vi "UHR-Fleezers Control (fpga) - 11.7.1UCBMeng4RG3.vi"() -> ()   [LabVIEW 2014]
doc: "UHR-Fleezers Instrument Control Code (fpga)"
uses:
  <vilib>/Platform/TimedLoop/XDataNode/timing_clust.ctl
  <vilib>/Platform/TimedLoop/XDataNode/nitl_modes.ctl
  <vilib>/Platform/TimedLoop/XDataNode/wakeup.ctl
  <vilib>/rvi/Emulation/niFpgaGetClockAttributes.vi
  <vilib>/rvi/Emulation/niFpgaSctlEmulationGetInTimedLoop.vi
  <vilib>/rvi/Emulation/niFpgaEmulationReportErrorSimple.vi
  <vilib>/rvi/Emulation/niFpgaProcessEmulError.vi
  <vilib>/rvi/eio/common/nirviEmuTemplateMethod_errors.vi
  <vilib>/rvi/Emulation/niFpgaCriticalErrorInLSC.vi
  <vilib>/rvi/interface/RandomDataEmulation/niFpgaRandomDataHandleErrors.vi
  <vilib>/eio/EIONode/EIONode.xnode
  <vilib>/eio/EIOMethodNode/EIOMethodNode.xnode
  <vilib>/rvi/DataTransferAndStorage/Container/XNode/niFpgaContainer.xnode
  <vilib>/rvi/interface/RandomDataEmulation/nirviRandomDataFpgaReadWriteTemplate.vi
  <vilib>/addons/control/pid/fpga.llb/XNode/niFpgaPID.xnode
  <vilib>/Platform/TimedLoop/XDataNode/XDataNode.xnode
  <vilib>/Platform/TimedLoop/XDataNode/XDNodeRunTimeDep.lvlib
panel:
  in  "Tab Control":T1(tab)=enum."Force FB"
  in  "Set 3":bool
  in  "Set 2":bool=TRUE
  in  "Set 1":bool=TRUE
  in  "Trap Pos to FIFO":bool
  in  "N of AI1 Int Acq Sets":i16=2 min=1 max=3 step=1
  out "AI Late Counter":u8
  in  "ai count":u16=400
  in  "+ phase":bool
  in  "Phase count adjustment":i16
  out "Relative phase":i16
  in  "AI to FIFO":bool
  out "BD1 Frequency Out 1":u64
  out "BD1 Frequency Out 2":u64
  out "Trap Pos FIFO Timeout":u16
  out "Trap AI FIFO Timeout":u16
  in  "Trap FIFO Set Timeout":i32
  in  "Tab Control 2":T2(tab)
  in  "FB Offset":u16
  in  "FB Multi Factor":i16
  in  "Dynamic FB (Ronen)":bool
  in  "Negate Intensity FB":bool
  in  "RD":bool
  in  "FB1 output high":i16=3000
  in  "FB1 output low":i16
  in  "D1":i16
  in  "I1":i16=5
  in  "P1":i16=10
  in  "Swap F1 and F2":bool
  in  "Cont. Scan":bool
  in  "Abort scan":bool
  in  "Cycles per step":u64
  in  "Scan BD":bool
  in  "Number of scans":u16
  in  "Scan steps":u64
  in  "Scan freq.  increment":i64
  out "Scanning":bool
  in  "Start scan":bool
  in  "OSK Bd 1":bool
  in  "Reset Bd 1":bool
  in  "PMODE":bool
  in  "Direct RF Box \nCommunication":bool
  in  "Data BD 2":u8 format="%08b"
  in  "Data BD 1":u8 format="%08b"
  in  "Address":u8 format="%02x"
  in  "Update Data":bool
  in  "FPGA Controls\n RF Box":bool
  in  "Number Interlace Cycles":u8=2 min=1 max=3
  in  "Interlace Off Parameters":u8=1 min=1 max=3
  in  "Interlace ON/OFF":bool
  out "DIO Relative phase":i16
  in  "Phase count adjustment (DIO)":i16
  in  "+ phase (DIO)":bool
  out "DIO Late Counter":u8
  in  "DIO count 1 (ticks)":u16=400
  in  "DIO count 2 (ticks)":u16=400
  in  "DIO count 3 (ticks)":u16=400
  out "AI2 Y Sum Set 2":i16
  out "AI2 Y Sum Set 1":i16
  in  "FB Setpoint Set 1":i16 min=0 step=1
  in  "FB Reset Set 1":bool
  in  "FB On/Off Set 1":bool
  in  "FB Reset Set 2":bool
  in  "FB On/Off Set 2":bool
  in  "FB Setpoint Set 2":i16 min=0 step=1
  out "Scan I":u64
  in  "Amp switch delay":u8=5
  in  "XY phase ext loop method":bool
  in  "BD 2 Amplitude 1":u16
  in  "BD 1 Amplitude 1":u16
  in  "BD 2 Frequency 1":u64
  in  "BD 1 Frequency 1":u64
  in  "BD 2 Amplitude 2":u16
  in  "BD 1 Amplitude 2":u16
  in  "BD 2 Frequency 2":u64
  in  "BD 1 Frequency 2":u64
  in  "BD 2 Amplitude 3":u16
  in  "BD 1 Amplitude 3":u16
  in  "BD 2 Frequency 3":u64
  in  "BD 1 Frequency 3":u64
  in  "BD 1 Delay (ticks)":u8
  in  "BD 2 Delay (Ticks)":u8 caption="Count(Ticks)"
  in  "Next trap write delay (ticks)":u8 caption="Count(Ticks)"
  in  "Trap 1 osc enable":bool
  in  "Trap 2 osc enable":bool
  in  "FB Min frequency":u64
  in  "FB Max Frequency":u64
  in  "Dynamic Force FB (Ronen)":bool
  in  "FB2 output high":fxp<+/-,16,1>=0.999969482421875
  in  "FB2 output low":fxp<+/-,16,1>=-1.0
  in  "P2":fxp<+/-,16,8> format="%.11g"
  in  "I2":fxp<+/-,16,8>=10.0 format="%.11g"
  in  "D2":fxp<+/-,16,8> format="%.11g"
  in  "Negate Diff?":bool
  in  "Diff FB Measurement?":bool
  in  "FB Trig Integrate":u32=1
  out "TTrig?":bool
  in  "TTrig Negate Pos":bool=TRUE
  out "Trap Pos FB Int Signal":fxp<+/-,24,9> format="%.18g"
  out "Trap Pos FB Int-Norm Signal":fxp<+/-,16,1> format="%.16g"
  in  "FPGA TTrig Thresh":i64
  in  "FPGA Trap Trig":bool
  out "Trap Pos FB Action":i64
  in  "Trap Pos. FB Offset Factor":i64
  in  "Trap Pos. FB Mult Factor":i64=2
  in  "Trap Pos. FB Reset":bool
  in  "Trap Pos FB Monitor T1 or T2":bool
  in  "AI1 X Scale":u16
  in  "Trap Pos FB Int Count":u16=100
  in  "Trap Pos FB Negate Action":bool
  out "AI1 X Set 2":fxp<+/-,16,1>
  out "AI1 X Set 1":fxp<+/-,16,1>
  in  "Trap Pos. FB SP":fxp<+/-,16,1>
  in  "Force feedback":bool
  out "TTrig Sig":i64
  out "TTrig Fin Thresh":i64
  in  "1D or 2D Scan?":bool
  in  "Abort scan (MCL)":bool
  in  "MCL Scan Axis":bool
  in  "Cont. Scan (MCL)":bool
  out "Scan I (MCL)":u64
  in  "Number of scans (MCL)":u16
  out "Scanning MCL":bool
  in  "Scan steps (MCL)":u64
  in  "Cycles per step (MCL)":u64
  in  "Scan freq.  increment (MCL)":i16
  in  "Start scan (MCL)":bool
  in  "AO2":i16
  in  "AO1":i16
  out "MCL Late Counter":u8
  in  "MCL count":u32=800
  out "MCL Relative Phase":i16
  in  "Phase count adjustment (MCL)":i16
  in  "+ phase (MCL)":bool
  out "APD2 int gate":bool
  out "APD3 out state":bool
  in  "APD Gate Operating Mode":u8 max=2 step=1
  in  "Invert APD Gate":bool
  in  "APD Gate OFF Count":u16=100
  in  "APD Gate ON Count":u16=300
  out "APD 1 Gate Late Counter":u8
  out "APD 1 Gate Relative Phase":i16
  in  "Phase count adjustment (APD 1 Gate)":i16
  in  "+ phase (APD 1 Gate)":bool
  out "APD 2 Counts 0":u32
  out "APD 2 Counts 1":u32
  out "APD 1 Counts 0":u32
  out "APD 1 Counts 1":u32
  out "APD1 out state":bool
  in  "APD AO scale factor":i16=1
  in  "APD to FIFO":bool
  in  "APD Acq Rate Count":u32=20000000
  out "APD Acq Late Counter":u8
  out "APD Acq Relative Phase":i16
  in  "Phase Count Adjustment (APD Acq)":i16
  in  "+ phase (APD Acq)":bool
  in  "Phase count adjustment (APD 2 Gate)":i16
  out "APD 2 Gate Late Counter":u8
  out "APD 2 Gate Relative Phase":i16
  in  "+ phase (APD 2 Gate)":bool
  out "APD2 out state":bool
  out "APD 3 Counts 0":u32
  out "APD 3 Counts 1":u32
  out "APD 3 Gate Late Counter":u8
  in  "Phase count adjustment (APD 3 Gate)":i16
  out "APD 3 Gate Relative Phase":i16
  in  "+ phase (APD 3 Gate)":bool
  out "APD1 int gate":bool
  out "APD3 int gate":bool
  in  "D3":i16
  in  "I3":i16=5
  in  "P3":i16=10
  in  "Green Filter Flipper":bool
  in  "Green FB Count":u16=1200
  out "Green Late Counter":u8
  out "Green FB Relative Phase":i16
  in  "Phase count adjustment (Green FB)":i16=10
  in  "+ phase (Green FB)":bool
  out "Green FB Sum":i16
  in  "Green int current ON count adj":u16=150
  in  "Current Out":u16=30000
  in  "Green FB On/Off":bool
  in  "Green FB Setpoint":i16=250 min=0 step=1
  in  "Green FB Reset":bool
  in  "Operating Mode 2":u8=2 max=2 step=1
  in  "Invert GI 2":bool
  in  "Green interlace OFF count 2":u16=900
  in  "Green interlace ON count 2":u16=300
  out "GI Late Counter 2":u8
  out "GI Relative phase 2":i16
  in  "Phase count adjustment (GI) 2":i16=20
  in  "+ phase (GI) 2":bool
  in  "Green interlace OFF count":u16=100
  out "GI Relative phase":i16
  in  "Phase count adjustment (GI)":i16
  in  "+ phase (GI)":bool
  in  "Green interlace ON count":u16=300
  out "GI Late Counter":u8
  in  "Invert GI":bool
  in  "Operating Mode":u8 max=2 step=1
  in  "+ phase (RI)":bool
  out "RI Relative phase":i16
  out "RI Late Counter":u8
  in  "Red interlace ON count":u16=300
  in  "Red interlace OFF count":u16=100
  in  "Invert RI":bool
  in  "Red Laser Operating Mode":u8 max=2 step=1
  in  "Phase count adjustment (RI)":i16
  out "Red FB Intensity":i16
  in  "RI Current Out":u16=30000
  in  "Red FB On/Off":bool
  in  "D4":i16
  in  "I4":i16=5
  in  "P4":i16=10
  in  "Red FB Setpoint":i16=250 min=0 step=1
  in  "Red FB Reset":bool
  in  "RI Operating Mode 2":u8=2 max=2 step=1
  in  "Invert RI 2":bool
  in  "Phase count adjustment (BI AO)":i16=20
  in  "Blue current ON count adj (AO)":u16=150
  in  "BI Current Out":i16=30000
  in  "Blue FB On/Off":bool
  in  "D5":i16
  in  "I5":i16=5
  in  "P5":i16=10
  in  "Blue FB Setpoint":i16=250 min=0 step=1
  in  "Blue FB Reset":bool
  in  "BI Operating Mode (AO)":u8=2 max=2 step=1
  in  "Invert BI (AO)":bool
  in  "Blue OFF count (AO)":u16=900
  in  "Blue ON count (AO)":u16=300
  out "BI Late Counter (AO)":u8
  out "BI Relative phase (AO)":i16
  in  "+ phase (BI AO)":bool
  in  "Phase count adjustment (BI D)":i16
  in  "Blue Laser Operating Mode (D)":u8 max=2 step=1
  in  "Invert BI (D)":bool
  in  "Blue interlace OFF count (D)":u16=100
  in  "Blue interlace ON count (D)":u16=300
  out "Blue Late Counter (D)":u8
  out "BI Relative phase (D)":i16
  in  "+ phase (BI D)":bool
  out "Blue Intensity":i16
  # "Only one of these can be on\nat a time:"
  # "Raster Scan AOD"
  # "1 (X)"
  # "2 (Y)"
  # "IR Intensity Feedback (RF BD 1)"
  # "FB Gains Set 1"
  # "FB output range 1"
  # "False is usual, True is external loop method"
  # "Parameters if using the external RF switching loop"
  # "Parameters if using the usual internal RF switching method"
  # "FB Triggering Excitation Laser"
  # "Trap Pos. FB Gains"
  # "Trap Pos. FB Range"
  # "AO1 (Y)"
  # "2D"
  # "1D"
  # "AO2 (X)"
  # "APD AO for aligning"
  # "Detection Loop"
  # "Green fluorescent laser digital gate interlacing loop"
  # "0 Forced ON\n1 Forced OFF\n2 Interlacing"
  # "Green FB Gains"
  # "Red fluorescent laser digital gate interlacing loop"
  # "Detection Loop"
  # "0 Forced ON\n1 Forced OFF\n2 Interlacing"
  # "Analog/FB Control Loop\n(Disabled)"
  # "Digital Control Loop"
  # "Blue laser intensity reading"
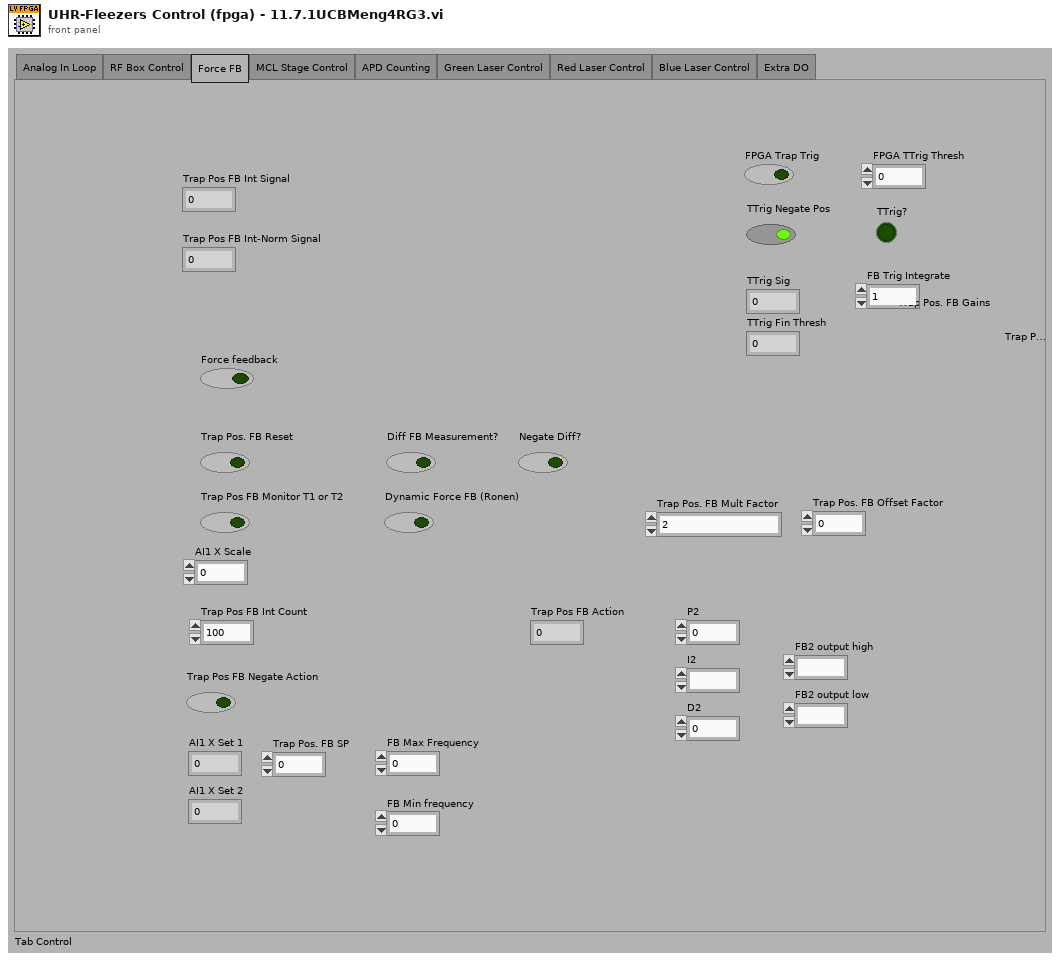
[diagram p1: front panel]
types:
  T1 = enum32{"Analog In Loop", "RF Box Control", "Force FB", "MCL Stage Control", "APD Counting", "Green Laser Control", "Red Laser Control", "Blue Laser Control", "Extra DO"}
  T2 = enum32{"Controls", "Interlacing Frequency and Amplitude Values", "Oscillate trap from memory"}
  T3 = typedef "XDNodeRunTimeDep.lvlib/timing_clust.ctl" = cluster{"Expected End [f-1]":u64, "Actual End [f-1]":u64, "Finished Late? [f-1]":bool, "Expected End [i-1]":u64, "Actual End [i-1]":u64, "Finished Late? [i-1]":bool, "Expected Start [i]":u64, "Actual Start [i]":u64, "Expected Start [f]":u64, "Actual Start [f]":u64, "Source Name":string, "Structure Name":string, "Period":i64, "Deadline":i64, "Offset":i64, "Start":i64, "Priority":i32, "Timeout":i32, "Mode":T4, "Wakeup Reason":T5, "Error":errorcluster, "Source Type":string, "Secondary Source Type":string, "Global End Time":u64, "Global Start Time":u64, "Frame Duration":u64, "Iteration Duration":u64, "Assigned CPU":i32, "I/O Scan Engine Mode":u32}
  T4 = typedef "XDNodeRunTimeDep.lvlib/nitl_modes.ctl" = enum32{"No Change", "Process missed periods, maintain original phase", "Discard missed periods, maintain original phase", "Process missed periods, ignore original phase", "Discard missed periods, ignore original phase"}
  T5 = typedef "XDNodeRunTimeDep.lvlib/wakeup.ctl" = enum32{"Normal", "Aborted", "Asynchronous wakeup", "Timing source error", "Timed loop error", "Timeout"}
  T6 = cluster{"proportional gain (Kc)":i16, "integral gain (Kc*Ts/Ti)":i16, "derivative gain (Kc*Td/Ts)":i16}
  T7 = cluster{"FB1 output high":i16, "FB1 output low":i16}
  T8 = cluster{"P2":fxp<+/-,16,8>, "I2":fxp<+/-,16,8>, "D2":fxp<+/-,16,8>}
  T9 = cluster{"FB2 output high":fxp<+/-,16,1>, "FB2 output low":fxp<+/-,16,1>}
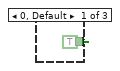
[diagram p2: hidden frame]
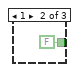
[diagram p3: hidden frame]
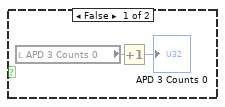
[diagram p6: hidden frame]
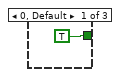
[diagram p8: hidden frame]
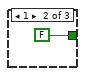
[diagram p9: hidden frame]
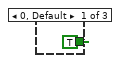
[diagram p10: hidden frame]
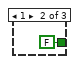
[diagram p11: hidden frame]
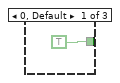
[diagram p13: hidden frame]
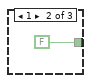
[diagram p14: hidden frame]
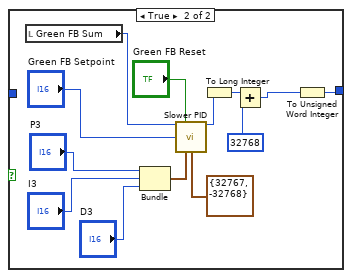
[diagram p17: hidden frame]
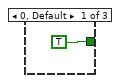
[diagram p18: hidden frame]
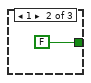
[diagram p19: hidden frame]
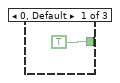
[diagram p20: hidden frame]
diagram:
  w6 = u16 0
  w7 = FALSE
  w5 = FALSE
  # "timing array current index"
  # "timing array"
  # "timing counter (phase adjusted here)"
  # "late counter"
  n1 = flat-sequence "FPGA initialization to do before running any of the loops" {
    tunnel: [u16 0 ("DIO count 3 (ticks)")] -> w4
    tunnel: [w15] -> _
    frame #0 {
      w14 = FALSE ("Enable")
      # "BD 2 (Y)"
      # "BD 1 (X)"
      # "Start up expansion chassis early\nto avoid delays later"
      # "This pin controls udclk on the RF boards.\nWhen initially configuring the boards, this pin needs to be\nconfigured as a high impedance input.  Later it will be switched\nto an output."
      # "Initial setting of DIO data and \naddress to low (before reset).  \nThis needs to happen before the other\ncontrol method loops execute."
      n2 = xnode "FPGA I/O Node"("Chassis2/Mod1/AO0"=u16 0 ("Chassis2/Mod4/AO0")) -> ("Chassis2/Mod2/AI0"=w15:i16)  [unwired: 2 in, 2 out]
      n3 = xnode "FPGA I/O Method Node"("Enable"=w14) -> ()  [unwired: 1 in, 1 out]
      n4 = xnode "FPGA I/O Method Node"("Enable"=w14) -> ()  [unwired: 1 in, 1 out]
      n5 = xnode "FPGA I/O Node"("Connector1/DIO0"=FALSE, "Connector1/DIO1"=FALSE, "Connector1/DIO2"=FALSE, "Connector1/DIO3"=FALSE, "Connector1/DIO4"=FALSE, "Connector1/DIO5"=FALSE, "Connector1/DIO6"=FALSE, "Connector1/DIO7"=FALSE, "Connector1/DIO8"=FALSE, "Connector1/DIO9"=FALSE, "Connector1/DIO10"=FALSE, "Connector1/DIO11"=FALSE, "Connector1/DIO12"=FALSE, "Connector1/DIO13"=FALSE, "Connector1/DIO15"=FALSE, "Connector1/DIO20"=FALSE, "Connector1/DIO21"=FALSE, "Connector1/DIO22"=FALSE, "Connector1/DIO23"=FALSE, "Connector1/DIO24"=FALSE, "Connector1/DIO25"=FALSE, "Connector1/DIO26"=FALSE, "Connector1/DIO27"=FALSE, "Connector1/DIO14"=FALSE) -> ()  [unwired: 24 in, 24 out]
    }
  }
  n6 = local read "AO1"() -> (w12:i16)
  n7 = local read "AO2"() -> (w11:i16)
  n8 = node-c288() -> (w10:T3)  [unwired: 1 in]
  n9 = disable-structure shown="Disabled" {
    disable-tunnel: w4 -> [w42 _]
    frame Disabled {
      n10 = while "Excitation laser intensity feedback measurement (all lasers)" {
        shift-right: [w43] -> _
        shift-left: w42 -> [w48]
        stop <- FALSE stop-if-true
        n11 = flat-sequence {
          tunnel: w48 -> [w50]
          tunnel: [w51] -> w46
          tunnel: [w50] -> w44
          tunnel: [w57] -> w47
          tunnel: w46 -> [w57]
          tunnel: [w56] -> w45
          tunnel: w44 -> [w56]
          tunnel: [w69] -> w43
          tunnel: w47 -> [w80]
          tunnel: w45 -> [w77]
          frame #0 {
            n12 = call "Loop Timer9"("Count(Ticks)"=w50) -> ("Tick Count(Ticks)"=w51:u16)
          }
          frame #1 {
            # "Design note:\n\nAll lasers need to be measured at the same \ntime because the AI expansion module\ncannot independently time the measurements\nwithin our requirements: their is dead time.\n\nThis probably wouldn't be an issue with the built\nin AI on the fpga board itself."
            n13 = xnode "FPGA I/O Node"("Connector1/DIO35"=TRUE) -> ("Chassis2/Mod2/AI2"=→"Blue Intensity":i16, "Chassis2/Mod2/AI1"=→"Red FB Intensity":i16, "Chassis2/Mod2/AI0"=→"Green FB Sum":i16)  [unwired: 4 in, 4 out]
          }
          frame #2 {
            n14 = feedback-in #1(w80) -> ()
            n15 = feedback #1(w80) -> (w79:u16)
            n16 = Subtract(x=w80, y=w79) -> (x-y=w78:u16)
            n17 = xnode "FPGA I/O Node"("Connector1/DIO35"=FALSE) -> ()  [unwired: 1 in, 1 out]
            n18 = Subtract(x=w78, y=w77) -> (x-y=w59:u16)
            n19 = Subtract(x="Green FB Count", y=w59) -> (x-y=w73:u16)
            n20 = Number To Boolean Array(number=w59) -> (Boolean array=w60:bool[])
            n21 = Or Array Elements(Boolean array=w60) -> (logical OR=w58:bool)
            n22 = Boolean To (0,1)(Boolean="+ phase (Green FB)") -> (0, 1=w71:i16)
            n23 = Boolean To (0,1)(Boolean=w58) -> (0, 1=w65:i16)
            n24 = Multiply(x=w71, y="Phase count adjustment (Green FB)") -> (x*y=w66:i16)
            n25 = Add(x=w73, y=w66) -> (x+y=w69:u16)
            n26 = To Unsigned Byte Integer(number=w65) -> (unsigned 8bit integer=w62:u8)
            n27 = feedback #2(i16 0) -> (w68:i16)
            n28 = Subtract(x=w68, y=w66) -> (x-y=w67:i16)
            "Green FB Relative Phase" <- w67
            n29 = feedback-in #2(w67) -> ()
            n30 = feedback #3(u8 0) -> (w63:u8)
            n31 = Add(x=w62, y=w63) -> (x+y=w61:u8)
            "Green Late Counter" <- w61
            n32 = feedback-in #3(w61) -> ()
          }
        }
      }
    }
    frame Enabled {
    }
  }
  n33 = To Unsigned Long Integer(number=w4) -> (unsigned 32bit integer=w8:u32)
  n34 = timed-loop "RF box board DIO control: control bits" {
    timing: w10 -> [_]
    timing-out: [_] -> w9
    tunnel: [w83] -> _
    tunnel: w4 -> [w83]
    stop <- FALSE stop-if-true
    n35 = xnode "FPGA I/O Node"("Connector1/DIO16"="RD", "Connector1/DIO17"="PMODE", "Connector1/DIO18"="OSK Bd 1", "Connector1/DIO19"="Reset Bd 1", "Connector0/DIO3"="Green Filter Flipper") -> ()  [unwired: 5 in, 5 out]
  }
  n36 = while "RF box board direct communication loop" {
    tunnel: w4 -> [_]
    stop <- FALSE stop-if-true
    n37 = case "Whether to use direct communication method (only use one method at a time)" shown="True" "Direct RF Box \nCommunication" {
      frame False {
      }
      frame True {
        n38 = case shown="True" "Update Data" {
          frame False {
          }
          frame True {
            n39 = flat-sequence {
              frame #0 {
                n40 = First Call?() -> (First Call?: T/F=w93:bool)
                n41 = case shown="True" w93 {
                  frame False {
                  }
                  frame True {
                    # "If first time data updated, be sure to set WR high\nbefore setting data and address bits."
                    n42 = flat-sequence {
                      frame #0 {
                        n43 = xnode "FPGA I/O Node"("Connector1/DIO15"=TRUE) -> ()  [unwired: 1 in, 1 out]
                      }
                      frame #1 {
                        n44 = call "Wait"("Count(Ticks)"=u8 40 ("DO Delay 3 (Ticks)")) -> ()  [unwired: 1 out]
                      }
                    }
                  }
                }
              }
              frame #1 {
                n45 = Number To Boolean Array(number="Address") -> (Boolean array=w142:bool[])
                n46 = Number To Boolean Array(number="Data BD 1") -> (Boolean array=w143:bool[])
                n47 = Number To Boolean Array(number="Data BD 2") -> (Boolean array=w112:bool[])
                n48 = Index Array(array=w143, index=7) -> (element=w127:bool)
                n49 = Index Array(array=w143, index=6) -> (element=w126:bool)
                n50 = Index Array(array=w143, index=5) -> (element=w125:bool)
                n51 = Index Array(array=w143, index=4) -> (element=w124:bool)
                n52 = Index Array(array=w143, index=3) -> (element=w123:bool)
                n53 = Index Array(array=w143, index=2) -> (element=w122:bool)
                n54 = Index Array(array=w143, index=1) -> (element=w121:bool)
                n55 = Index Array(array=w143, index=0) -> (element=w120:bool)
                n56 = Index Array(array=w142, index=5) -> (element=w119:bool)
                n57 = Index Array(array=w142, index=4) -> (element=w118:bool)
                n58 = Index Array(array=w142, index=3) -> (element=w117:bool)
                n59 = Index Array(array=w142, index=2) -> (element=w116:bool)
                n60 = Index Array(array=w142, index=1) -> (element=w115:bool)
                n61 = Index Array(array=w142, index=0) -> (element=w114:bool)
                n62 = Index Array(array=w112, index=7) -> (element=w103:bool)
                n63 = Index Array(array=w112, index=6) -> (element=w102:bool)
                n64 = Index Array(array=w112, index=5) -> (element=w101:bool)
                n65 = Index Array(array=w112, index=4) -> (element=w100:bool)
                n66 = Index Array(array=w112, index=3) -> (element=w99:bool)
                n67 = Index Array(array=w112, index=2) -> (element=w98:bool)
                n68 = Index Array(array=w112, index=1) -> (element=w97:bool)
                n69 = Index Array(array=w112, index=0) -> (element=w96:bool)
                n70 = xnode "FPGA I/O Node"("Connector1/DIO0"=w127, "Connector1/DIO1"=w126, "Connector1/DIO2"=w125, "Connector1/DIO3"=w124, "Connector1/DIO4"=w123, "Connector1/DIO5"=w122, "Connector1/DIO6"=w121, "Connector1/DIO7"=w120, "Connector1/DIO8"=w119, "Connector1/DIO9"=w118, "Connector1/DIO10"=w117, "Connector1/DIO11"=w116, "Connector1/DIO12"=w115, "Connector1/DIO13"=w114, "Connector1/DIO20"=w103, "Connector1/DIO21"=w102, "Connector1/DIO22"=w101, "Connector1/DIO23"=w100, "Connector1/DIO24"=w99, "Connector1/DIO25"=w98, "Connector1/DIO26"=w97, "Connector1/DIO27"=w96) -> ()  [unwired: 22 in, 22 out]
              }
              frame #2 {
                # "wait and then apply write signal"
                n71 = call "Wait2"("Count(Ticks)"=u8 40 ("DO Delay 1 (Ticks)")) -> ()  [unwired: 1 out]
              }
              frame #3 {
                # "sending bit low writes data to board buffer"
                n72 = xnode "FPGA I/O Node"("Connector1/DIO15"=FALSE) -> ()  [unwired: 1 in, 1 out]
              }
              frame #4 {
                # "wait then return write signal"
                n73 = call "Wait3"("Count(Ticks)"=u8 40 ("DO Delay 2 (Ticks)")) -> ()  [unwired: 1 out]
              }
              frame #5 {
                # "sending bit high makes ready to\nwrite more data"
                n74 = xnode "FPGA I/O Node"("Connector1/DIO15"=TRUE) -> ()  [unwired: 1 in, 1 out]
              }
            }
          }
        }
      }
    }
  }
  n75 = while "RF box board DIO control: parallel communication" {
    shift-right: [w162] -> _
    shift-left: w4 -> [w161]
    shift-right: [w160] -> _
    shift-left: FALSE ("Swap F1 and F2") -> [w159]
    shift-right: [w154] -> _
    shift-left: u16 0 -> [w155]
    shift-right: [w152] -> _
    shift-left: u16 0 -> [w153]
    shift-right: [w150] -> _
    shift-left: u64 0 -> [w151]
    stop <- FALSE stop-if-true
    n76 = flat-sequence {
      tunnel: w159 -> [w166]
      tunnel: w161 -> [w164]
      tunnel: [w166] -> w158
      tunnel: [w165] -> w157
      tunnel: [w164] -> w156
      tunnel: [w178] -> w162
      tunnel: [w177] -> w160
      tunnel: w158 -> [w176]
      tunnel: w157 -> [w174]
      tunnel: w156 -> [w173]
      tunnel: w155 -> [w172]
      tunnel: [w171] -> w154
      tunnel: w153 -> [w170]
      tunnel: [w169] -> w152
      tunnel: w151 -> [w168]
      tunnel: [w167] -> w150
      frame #0 {
        n77 = call "Loop Timer"("Count(Ticks)"=w164) -> ("Tick Count(Ticks)"=w165:u16)
      }
      frame #1 {
        n78 = flat-sequence {
          tunnel: ["FPGA Controls\n RF Box"] -> w175
          tunnel: w176 -> [w179]
          tunnel: [w242] -> w178
          tunnel: [w255] -> w177
          tunnel: w175 -> [w254]
          tunnel: w174 -> [w248]
          tunnel: w173 -> [w245]
          tunnel: w172 -> [w211]
          tunnel: [w210] -> w171
          tunnel: w170 -> [w207]
          tunnel: [w206] -> w169
          tunnel: w168 -> [w205]
          tunnel: [w204] -> w167
          frame #0 {
            n79 = case shown="True" "FPGA Controls\n RF Box" {
              tunnel: w179 -> [_ w181]
              frame False {
              }
              frame True {
                n80 = flat-sequence {
                  tunnel: w181 -> [w191]
                  frame #0 {
                    n81 = First Call?() -> (First Call?: T/F=w182:bool)
                    n82 = case shown="True" w182 {
                      frame False {
                      }
                      frame True {
                        # "BD 2"
                        # "BD 1"
                        # "If first time data updated, be sure to set WR high and UDCLK low\nbefore setting data and address bits."
                        n83 = xnode "FPGA I/O Method Node"("Enable"=TRUE) -> ("FPGA I/O Out"=w184:refnum<k21>)  [unwired: 1 in]
                        n84 = xnode "FPGA I/O Method Node"("Enable"=TRUE) -> ("FPGA I/O Out"=w187:refnum<k21>)  [unwired: 1 in]
                        n85 = xnode "FPGA I/O Node"("Connector1/DIO15"=TRUE) -> ()  [unwired: 1 in, 1 out]
                        n86 = xnode "FPGA I/O Node"("I/O Item"=FALSE ("Connector1/DIO30"), "FPGA I/O In"=w184) -> ()  [unwired: 1 out]
                        n87 = xnode "FPGA I/O Node"("I/O Item"=FALSE ("Connector1/DIO30"), "FPGA I/O In"=w187) -> ()  [unwired: 1 out]
                      }
                    }
                  }
                  frame #1 {
                    n88 = case shown="False" FALSE {
                      tunnel: w191 -> [w193 _]
                      frame False {
                        # "Usual operation"
                        n89 = flat-sequence "BD 1 (X)" {
                          tunnel: w193 -> [w200]
                          tunnel: "Amp switch delay" -> [w201]
                          frame #0 {
                            n90 = call "Wait6"("Count(Ticks)"="BD 1 Delay (ticks)") -> ()  [unwired: 1 out]
                          }
                          frame #1 {
                            # "switch frequency"
                            n91 = xnode "FPGA I/O Node"("Connector1/DIO36"=w200) -> ()  [unwired: 1 in, 1 out]
                          }
                          frame #2 {
                            # "~5 ticks is usual"
                            n92 = call "Wait4"("Count(Ticks)"=w201) -> ()  [unwired: 1 out]
                          }
                          frame #3 {
                            # "this switches amplitude"
                            # "switch amplitude"
                            # "send udclk high"
                            n93 = xnode "FPGA I/O Node"("Connector1/DIO30"=TRUE ("Connector1/DIO15")) -> ()  [unwired: 1 in, 1 out]
                          }
                          frame #4 {
                            # "reset to be ready for next\ncycle"
                            # "send udclk low"
                            n94 = xnode "FPGA I/O Node"("Connector1/DIO30"=FALSE ("Connector1/DIO15")) -> ()  [unwired: 1 in, 1 out]
                          }
                        }
                        n95 = flat-sequence "BD 2 (Y)" {
                          tunnel: w193 -> [w195]
                          tunnel: "Amp switch delay" -> [w196]
                          frame #0 {
                            n96 = call "Wait7"("Count(Ticks)"="BD 2 Delay (Ticks)") -> ()  [unwired: 1 out]
                          }
                          frame #1 {
                            # "switch frequency"
                            n97 = xnode "FPGA I/O Node"("Connector1/DIO37"=w195) -> ()  [unwired: 1 in, 1 out]
                          }
                          frame #2 {
                            # "~5 ticks is usual"
                            n98 = call "Wait5"("Count(Ticks)"=w196) -> ()  [unwired: 1 out]
                          }
                          frame #3 {
                            # "this switches amplitude"
                            # "switch amplitude"
                            # "send udclk high"
                            n99 = xnode "FPGA I/O Node"("Connector1/DIO29"=TRUE ("Connector1/DIO15")) -> ()  [unwired: 1 in, 1 out]
                          }
                          frame #4 {
                            # "reset to be ready for next\ncycle"
                            # "send udclk low"
                            n100 = xnode "FPGA I/O Node"("Connector1/DIO29"=FALSE ("Connector1/DIO15")) -> ()  [unwired: 1 in, 1 out]
                          }
                        }
                      }
                      frame True {
                        # "Operation when you need a long delay for either X or Y to synchonize AOD light out phase (> ~100 ticks)."
                        # "Trigger the external loop by sending the boolean FSK value through a FIFO"
                      }
                    }
                  }
                }
              }
            }
          }
          frame #1 {
            # "This is the prior cycle's on time"
            # "increment timing\nindex, reset to 0 if \nend of matrix"
            # "Reset to begginning (1) when number of cycles reached."
            # "timing index"
            # "build byte stacks for writing data\n(must correspond to addresses array constant)"
            # "Timing housekeeping"
            # "Adjust phase if late\n(maintains constant phase relationship between cycles)"
            n101 = Bundle("FB1 output high"="FB1 output high", "FB1 output low"="FB1 output low") -> (w215:T7)  [unwired: 1 in]
            n102 = Bundle("P1"="P1", "I1"="I1", "D1"="D1") -> (w216:cluster{"P1":i16, "I1":i16, "D1":i16})  [unwired: 1 in]
            n103 = feedback #4(u8 0 ("t")) -> (w251:u8)
            n104 = Increment(x=w251) -> (x+1=w294:u8)
            n105 = Increment(x="Number Interlace Cycles") -> (x+1=w289:u8)
            n106 = Equal?(x=w294, y=w289) -> (x = y?=w296:bool)
            n107 = Select(t=u8 1, s=w296, f=w294) -> (s? t:f=w250:u8)
            n108 = feedback-in #4(w250) -> ()
            n109 = Increment(x=w250) -> (x+1=w291:u8)
            n110 = Equal?(x=w291, y=w289) -> (x = y?=w292:bool)
            n111 = Select(t=u8 1, s=w292, f=w291) -> (s? t:f=w288:u8)
            n112 = Select(t=w288, s="Interlace ON/OFF", f="Interlace Off Parameters") -> (s? t:f=w214:u8)
            n113 = case shown="1, Default" w214 {
              tunnel: [w335 w590 "BD 1 Frequency 3"] -> w284
              tunnel: [w385 "BD 2 Frequency 2" "BD 2 Frequency 3"] -> w273
              tunnel: ["BD 2 Amplitude 1" "BD 2 Amplitude 2" "BD 2 Amplitude 3"] -> w230
              tunnel: [w344 w584 "BD 1 Amplitude 3"] -> w233
              tunnel: w216 -> [w352 w592 _]
              tunnel: w215 -> [w353 w591 _]
              tunnel: "Negate Intensity FB" -> [w351 w588 _]
              tunnel: "Dynamic FB (Ronen)" -> [w350 w587 _]
              tunnel: w211 -> [w345 w586 w638]
              tunnel: [w344 w586 w638] -> w210
              tunnel: "FB Multi Factor" -> [w343 w583 _]
              tunnel: "FB Offset" -> [w342 w582 _]
              tunnel: w207 -> [w341 w585 w637]
              tunnel: [w341 w584 w637] -> w206
              tunnel: w205 -> [w340 w581 w636]
              tunnel: [w335 w581 w636] -> w204
              frame 1, Default {
                w368 = fxp<+/-,24,9> 0.0 ("AI1 X Set 2")
                w361 = u16 0
                w381 = u64 0 ("f")
                # "Added by Ronen -\nUpper and Lower \nLimits for the FB \ngenerated frequency\nto avoid losing bead \nwhen tether breaks"
                # "Changed by Ronen - correction \nby PID is now implemented not on \nthe Base BD1 frequency but on the last\nfrequency sent."
                # "BD1 Amp 1"
                # "Changed by Ronen-\n FB changed \nso that value from PID is added to\nlast amplitude sent to board. Correction\nValue can be scaled down same as the force\nFB value."
                # "This signal integration happens no matter what\nso that correct setpoints can be chosen before \nturning on the FB."
                # "Trap 1"
                n114 = local read "AI1 X Set 2"() -> (w364:fxp<+/-,16,1>)
                n115 = local read "AI1 X Set 1"() -> (w365:fxp<+/-,16,1>)
                n116 = local read "Scanning"() -> (w386:bool)
                n117 = Or(x=w386, y="Start scan") -> (x .or. y?=w379:bool)
                n118 = case shown="True" "Diff FB Measurement?" {
                  tunnel: w364 -> [w404 w413]
                  tunnel: w365 -> [w403 w414]
                  tunnel: [w401 w405] -> w366
                  frame False {
                    n119 = Select(t=w403, s="Trap Pos FB Monitor T1 or T2", f=w404) -> (s? t:f=w401:fxp<+/-,16,1>)
                  }
                  frame True {
                    n120 = Subtract(x=w414, y=w413) -> (x-y=w406:fxp<+/-,17,2>)
                    n121 = Not(x="Negate Diff?") -> (.not. x?=w412:bool)
                    n122 = Boolean To (0,1)(Boolean="Negate Diff?") -> (0, 1=w410:i16)
                    n123 = Boolean To (0,1)(Boolean=w412) -> (0, 1=w411:i16)
                    n124 = Negate(x=w410) -> (-x=w409:i16)
                    n125 = Add(x=w409, y=w411) -> (x+y=w407:i16)
                    n126 = Multiply(x=w407, y=w406) -> (x*y=w405:fxp<+/-,32,17>)
                  }
                }
                n127 = Not(x="Abort scan") -> (.not. x?=w377:bool)
                n128 = And(x=w377, y=w379) -> (x .and. y?=w376:bool)
                n129 = case "For raster scanning" shown="True" w376 {
                  tunnel: [u64 0 w540] -> w382
                  tunnel: "Start scan" -> [_ w525]
                  frame False {
                    n130 = local write "Scanning"(FALSE ("scanning")) -> ()
                  }
                  frame True {
                    w509 = i64 0
                    w508 = u64 0
                    # "scan incr."
                    # "freq. incr. mult."
                    # "count steps"
                    # "count number of cycles"
                    n131 = feedback #5(w508) -> (w537:u64)
                    n132 = Select(t=w508, s=w525, f=w537) -> (s? t:f=w539:u64)
                    n133 = Increment(x=w539) -> (x+1=w536:u64)
                    n134 = Greater?(x="Cycles per step", y=w536) -> (0:w518:bool)
                    n135 = Select(t=w536, s=w518, f=w508) -> (s? t:f=w535:u64)
                    n136 = feedback-in #5(w535) -> ()
                    n137 = feedback #6(w508) -> (w534:u64)
                    n138 = Select(t=w508, s=w525, f=w534) -> (s? t:f=w529:u64)
                    n139 = Increment(x=w529) -> (x+1=w533:u64)
                    n140 = Add(x="Scan steps", y="Scan steps") -> (x+y=w532:u64)
                    n141 = Select(t=w529, s=w518, f=w533) -> (s? t:f=w513:u64)
                    n142 = Greater?(x=w532, y=w513) -> (0:w512:bool)
                    n143 = Select(t=w513, s=w512, f=w508) -> (s? t:f=w530:u64)
                    n144 = feedback-in #6(w530) -> ()
                    n145 = Equal?(x="Scan steps", y=w513) -> (x = y?=w517:bool)
                    n146 = Greater?(x="Scan steps", y=w529) -> (0:w528:bool)
                    n147 = feedback #7(w509) -> (w531:i64)
                    n148 = Select(t=w509, s=w525, f=w531) -> (s? t:f=w515:i64)
                    n149 = Increment(x=w515) -> (x+1=w527:i64)
                    n150 = Decrement(x=w515) -> (x-1=w526:i64)
                    n151 = Select(t=w527, s=w528, f=w526) -> (s? t:f=w516:i64)
                    n152 = Select(t=w515, s=w517, f=w516) -> (s? t:f=w514:i64)
                    n153 = Select(t=w515, s=w518, f=w514) -> (s? t:f=w510:i64)
                    n154 = Select(t=w510, s=w512, f=w509) -> (s? t:f=w511:i64)
                    n155 = feedback-in #7(w511) -> ()
                    n156 = feedback #8(w508) -> (w524:u64)
                    n157 = Select(t=w508, s=w525, f=w524) -> (s? t:f=w520:u64)
                    n158 = Increment(x=w520) -> (x+1=w521:u64)
                    n159 = Select(t=w520, s=w512, f=w521) -> (s? t:f=w519:u64)
                    n160 = Greater?(x="Number of scans", y=w519) -> (0:w505:bool)
                    n161 = Multiply(x="Scan freq.  increment", y=w515) -> (x*y=w540:i64)
                    n162 = Select(t=TRUE, s="Cont. Scan", f=w505) -> (s? t:f=w504:bool)
                    "Scanning" <- w504
                    n163 = Select(t=w519, s=w504, f=w508) -> (s? t:f=w522:u64)
                    n164 = feedback-in #8(w522) -> ()
                    n165 = Increment(x=w519) -> (x+1=→"Scan I":u64)
                  }
                }
                n166 = feedback #9(w361) -> (w360:u16)
                n167 = Increment(x=w360) -> (x+1=w362:u16)
                n168 = Greater Or Equal?(x=w362, y="Trap Pos FB Int Count") -> (x >= y?=w339:bool)
                n169 = Select(t=w361, s=w339, f=w362) -> (s? t:f=w363:u16)
                n170 = feedback-in #9(w363) -> ()
                n171 = feedback #10(w368) -> (w367:fxp<+/-,24,9>)
                n172 = Add(x=w366, y=w367) -> (x+y=w359:fxp<+/-,24,9>)
                n173 = case "For intensity feedback" shown="True" "FB On/Off Set 1" {
                  tunnel: w345 -> [_ w545]
                  tunnel: ["BD 1 Amplitude 1" w551] -> w344
                  tunnel: w353 -> [_ w552]
                  tunnel: w352 -> [_ w553]
                  tunnel: w351 -> [_ w550]
                  tunnel: w350 -> [_ w549]
                  tunnel: w343 -> [_ w544]
                  tunnel: w342 -> [_ w543]
                  frame False {
                  }
                  frame True {
                    n174 = local read "AI2 Y Sum Set 1"() -> (w547:i16)
                    n175 = case shown="True" w549 {
                      tunnel: w553 -> [w559 w573]
                      tunnel: w552 -> [w560 w572]
                      tunnel: [w554 w571] -> w551
                      tunnel: w550 -> [_ w570]
                      tunnel: "FB Setpoint Set 1" -> [w558 w569]
                      tunnel: w547 -> [w557 w568]
                      tunnel: "FB Reset Set 1" -> [w556 w567]
                      tunnel: w545 -> [_ w566]
                      tunnel: w544 -> [_ w564]
                      tunnel: w543 -> [_ w562]
                      frame False {
                        n176 = call "Slower PID.vi"("process variable"=w557, "reset?"=w556, "setpoint"=w558, "PID gains (x 2^8)"=w559, "output range"=w560) -> ("output"=w555:i16)  [unwired: 10 out]
                        n177 = To Unsigned Word Integer(number=w555) -> (unsigned 16bit integer=w554:u16)
                      }
                      frame True {
                        n178 = call "Slower PID.vi"("process variable"=w568, "reset?"=w567, "setpoint"=w569, "PID gains (x 2^8)"=w573, "output range"=w572) -> ("output"=w574:i16)  [unwired: 10 out]
                        n179 = To Unsigned Word Integer(number=w574) -> (unsigned 16bit integer=w565:u16)
                        n180 = Scale By Power Of 2(n=w564, x=w565) -> (x*2^n=w563:u16)
                        n181 = Add(x=w563, y=w562) -> (x+y=w561:u16)
                        n182 = case shown="True" w570 {
                          tunnel: w561 -> [w577 w579]
                          tunnel: w566 -> [w575 w580]
                          tunnel: [w576 w578] -> w571
                          frame False {
                            n183 = Add(x=w575, y=w577) -> (x+y=w576:u16)
                          }
                          frame True {
                            n184 = Subtract(x=w580, y=w579) -> (x-y=w578:u16)
                          }
                        }
                      }
                    }
                  }
                }
                n185 = Select(t=w368, s=w339, f=w359) -> (s? t:f=w371:fxp<+/-,24,9>)
                n186 = feedback-in #10(w371) -> ()
                n187 = Divide(x=w359, y="Trap Pos FB Int Count") -> (x/y=w354:fxp<+/-,16,1>)
                n188 = feedback #11(fxp<+/-,24,9> 0.0 ("AI1 X Set 2")) -> (w372:fxp<+/-,24,9>)
                n189 = Select(t=w359, s=w339, f=w372) -> (s? t:f=w373:fxp<+/-,24,9>)
                "Trap Pos FB Int Signal" <- w373
                n190 = feedback-in #11(w373) -> ()
                n191 = feedback #12(fxp<+/-,16,1> 0.0 ("Trap Pos FB Int-Norm Signal")) -> (w356:fxp<+/-,16,1>)
                n192 = Select(t=w354, s=w339, f=w356) -> (s? t:f=w355:fxp<+/-,16,1>)
                "Trap Pos FB Int-Norm Signal" <- w355
                n193 = feedback-in #12(w355) -> ()
                n194 = case "For position feedback" shown="True" "Force feedback" {
                  tunnel: [i64 0 w420] -> w349
                  tunnel: w354 -> [_ w417]
                  tunnel: w339 -> [_ w416]
                  frame False {
                  }
                  frame True {
                    n195 = feedback #13(i64 0) -> (w419:i64)
                    n196 = case shown="True" w416 {
                      tunnel: [w421 w435] -> w420
                      tunnel: w419 -> [w421 _]
                      tunnel: w417 -> [_ w429]
                      frame False {
                      }
                      frame True {
                        w439 = u32 0
                        n197 = Bundle("P2"="P2", "I2"="I2", "D2"="D2") -> (w425:T8)  [unwired: 1 in]
                        n198 = Bundle("FB2 output high"="FB2 output high", "FB2 output low"="FB2 output low") -> (w422:T9)  [unwired: 1 in]
                        n199 = xnode ("PID")("process variable"=w429, "reset?"="Trap Pos. FB Reset", "setpoint"="Trap Pos. FB SP", "PID gains"=w425, "output range"=w422) -> ("output"=w451:fxp<+/-,16,1>)
                        n200 = Negate(x=w451) -> (-x=w450:fxp<+/-,17,2>)
                        n201 = Select(t=w450, s="Trap Pos FB Negate Action", f=w451) -> (s? t:f=w447:fxp<+/-,17,2>)
                        n202 = Scale By Power Of 2(n=u32 15, x=u32 1) -> (x*2^n=w444:u32)
                        n203 = Multiply(x=w447, y=w444) -> (x*y=w443:fxp<+/-,17,17>)
                        n204 = To Quad Integer(1:w443) -> (0:w455:i64)
                        "Trap Pos FB Action" <- w455
                        n205 = Multiply(x=w455, y="Trap Pos. FB Mult Factor") -> (x*y=w453:i64)
                        n206 = Add(x=w453, y="Trap Pos. FB Offset Factor") -> (x+y=w435:i64)
                        n207 = feedback #14() -> (w436:i64)  [unwired: 1 in]
                        n208 = Add(x=w435, y=w436) -> (x+y=w433:i64)
                        n209 = feedback #15(w439) -> (w441:u32)
                        n210 = Increment(x=w441) -> (x+1=w430:u32)
                        n211 = Greater Or Equal?(x=w430, y="FB Trig Integrate") -> (x >= y?=w431:bool)
                        n212 = Select(t=i64 0, s=w431, f=w433) -> (s? t:f=w437:i64)
                        n213 = feedback-in #14(w437) -> ()
                        n214 = Select(t=w439, s=w431, f=w430) -> (s? t:f=w440:u32)
                        n215 = feedback-in #15(w440) -> ()
                        n216 = And(x=w431, y="FPGA Trap Trig") -> (x .and. y?=w438:bool)
                        n217 = case "Trap FB trigger excitation laser ON" shown="True" w438 {
                          tunnel: w433 -> [_ w459]
                          tunnel: w430 -> [_ w457]
                          frame False {
                          }
                          frame True {
                            n218 = Not(x="TTrig Negate Pos") -> (.not. x?=w466:bool)
                            n219 = Boolean To (0,1)(Boolean="TTrig Negate Pos") -> (0, 1=w464:i16)
                            n220 = Boolean To (0,1)(Boolean=w466) -> (0, 1=w465:i16)
                            n221 = Negate(x=w464) -> (-x=w463:i16)
                            n222 = Add(x=w463, y=w465) -> (x+y=w462:i16)
                            n223 = Multiply(x=w462, y=w459) -> (x*y=w461:i64)
                            "TTrig Sig" <- w461
                            n224 = Multiply(x="FPGA TTrig Thresh", y=w457) -> (x*y=w458:i64)
                            "TTrig Fin Thresh" <- w458
                            n225 = Greater Or Equal?(x=w461, y=w458) -> (x >= y?=w460:bool)
                            n226 = case shown="True" w460 {
                              frame False {
                              }
                              frame True {
                                w469 = TRUE ("Green FB On/Off")
                                w471 = u8 2 ("Operating Mode")
                                n227 = local write "Operating Mode 2"(w471) -> ()
                                n228 = local write "Operating Mode"(w471) -> ()
                                n229 = local write "Green FB On/Off"(w469) -> ()
                                n230 = local write "FPGA Trap Trig"(FALSE ("FPGA Trap Trig")) -> ()
                                "TTrig?" <- w469
                              }
                            }
                          }
                        }
                      }
                    }
                    n231 = feedback-in #13(w420) -> ()
                  }
                }
                n232 = case shown="True" "Dynamic Force FB (Ronen)" {
                  tunnel: w349 -> [w392 w396]
                  tunnel: [w391 w395] -> w347
                  tunnel: w340 -> [_ w394]
                  tunnel: w339 -> [_ w393]
                  frame False {
                    # "(BD1 Frequency 1)"
                    n233 = Add(x="BD 1 Frequency 1", y=w392) -> (x+y=w391:u64)
                  }
                  frame True {
                    n234 = case shown="False" w393 {
                      tunnel: w396 -> [_ w400]
                      tunnel: [w397 w399] -> w395
                      tunnel: w394 -> [w397 w398]
                      frame False {
                      }
                      frame True {
                        n235 = Add(x=w398, y=w400) -> (x+y=w399:u64)
                      }
                    }
                  }
                }
                n236 = Select(t=w381, s="Scan BD", f=w382) -> (s? t:f=w380:u64)
                n237 = Select(t=w382, s="Scan BD", f=w381) -> (s? t:f=w383:u64)
                n238 = Add(x=w380, y="BD 2 Frequency 1") -> (x+y=w385:u64)
                n239 = Compound Arithmetic op=ADD(i64 0 ("f"), w347, w383) -> (w338:u64)
                "BD1 Frequency Out 1" <- w338
                n240 = In Range and Coerce(upper limit="FB Max Frequency", x=w338, lower limit="FB Min frequency") -> (coerced(x)=w335:u64)  [unwired: 1 out]
              }
              frame 2 {
                # "Trap 2"
                n241 = case shown="True" "FB On/Off Set 2" {
                  tunnel: ["BD 1 Amplitude 2" w602] -> w584
                  tunnel: w585 -> [_ w600]
                  tunnel: w592 -> [_ w605]
                  tunnel: w591 -> [_ w604]
                  tunnel: w588 -> [_ w603]
                  tunnel: w587 -> [_ w601]
                  tunnel: w583 -> [_ w599]
                  tunnel: w582 -> [_ w598]
                  frame False {
                  }
                  frame True {
                    n242 = local read "AI2 Y Sum Set 2"() -> (w607:i16)
                    n243 = case shown="False" w601 {
                      tunnel: "FB Setpoint Set 2" -> [w613 w629]
                      tunnel: w607 -> [w614 w628]
                      tunnel: "FB Reset Set 2" -> [w615 w627]
                      tunnel: w605 -> [w611 w625]
                      tunnel: w604 -> [w612 w624]
                      tunnel: w603 -> [_ w623]
                      tunnel: [w609 w622] -> w602
                      tunnel: w600 -> [_ w621]
                      tunnel: w599 -> [_ w620]
                      tunnel: w598 -> [_ w617]
                      frame False {
                        n244 = call "Slower PID.vi"("process variable"=w614, "reset?"=w615, "setpoint"=w613, "PID gains (x 2^8)"=w611, "output range"=w612) -> ("output"=w610:i16)  [unwired: 10 out]
                        n245 = To Unsigned Word Integer(number=w610) -> (unsigned 16bit integer=w609:u16)
                      }
                      frame True {
                        n246 = call "Slower PID.vi"("process variable"=w628, "reset?"=w627, "setpoint"=w629, "PID gains (x 2^8)"=w625, "output range"=w624) -> ("output"=w626:i16)  [unwired: 10 out]
                        n247 = To Unsigned Word Integer(number=w626) -> (unsigned 16bit integer=w619:u16)
                        n248 = Scale By Power Of 2(n=w620, x=w619) -> (x*2^n=w618:u16)
                        n249 = Add(x=w618, y=w617) -> (x+y=w616:u16)
                        n250 = case shown="False" w623 {
                          tunnel: w621 -> [w631 w635]
                          tunnel: w616 -> [w630 w634]
                          tunnel: [w632 w633] -> w622
                          frame False {
                            n251 = Add(x=w631, y=w630) -> (x+y=w632:u16)
                          }
                          frame True {
                            n252 = Subtract(x=w635, y=w634) -> (x-y=w633:u16)
                          }
                        }
                      }
                    }
                  }
                }
                n253 = Add(x="BD 1 Frequency 2", y=i64 0 ("f")) -> (x+y=w590:u64)
                "BD1 Frequency Out 2" <- w590
              }
              frame 3 {
                # "Fluorescence period"
              }
            }
            n254 = feedback-in #16(w248) -> ()
            n255 = feedback #16(w248) -> (w247:u16)
            n256 = Select(t=w250, s="Interlace ON/OFF", f="Interlace Off Parameters") -> (s? t:f=w287:u8)
            n257 = Subtract(x=w248, y=w247) -> (x-y=w246:u16)
            n258 = Subtract "The error"(x=w246, y=w245) -> (x-y=w223:u16)
            n259 = case shown="1, Default" w287 {
              tunnel: ["DIO count 1 (ticks)" "DIO count 2 (ticks)" "DIO count 3 (ticks)"] -> w244
              frame 1, Default {
              }
              frame 2 {
              }
              frame 3 {
              }
            }
            n260 = Number To Boolean Array(number=w223) -> (Boolean array=w224:bool[])
            n261 = Or Array Elements(Boolean array=w224) -> (logical OR=w222:bool)
            n262 = Boolean To (0,1)(Boolean=w222) -> (0, 1=w229:i16)
            n263 = To Unsigned Byte Integer(number=w229) -> (unsigned 8bit integer=w226:u8)
            n264 = feedback #17(u8 0) -> (w227:u8)
            n265 = Add(x=w226, y=w227) -> (x+y=w225:u8)
            "DIO Late Counter" <- w225
            n266 = feedback-in #17(w225) -> ()
            n267 = Subtract(x=w244, y=w223) -> (x-y=w243:u16)
            n268 = Split Number(x=w284) -> (hi(x)=w283:u32, lo(x)=w282:u32)
            n269 = Split Number(x=w273) -> (hi(x)=w278:u32, lo(x)=w277:u32)
            n270 = Boolean To (0,1)(Boolean="+ phase (DIO)") -> (0, 1=w240:i16)
            n271 = Split Number(x=w283) -> (lo(x)=w281:u16)  [unwired: 1 out]
            n272 = Split Number(x=w282) -> (hi(x)=w280:u16, lo(x)=w279:u16)
            n273 = Split Number(x=w278) -> (lo(x)=w276:u16)  [unwired: 1 out]
            n274 = Split Number(x=w277) -> (hi(x)=w275:u16, lo(x)=w274:u16)
            n275 = Split Number(x=w233) -> (hi(x)=w235:u8, lo(x)=w234:u8)
            n276 = Split Number(x=w230) -> (hi(x)=w232:u8, lo(x)=w231:u8)
            n277 = Split Number(x=w281) -> (hi(x)=w272:u8, lo(x)=w271:u8)
            n278 = Split Number(x=w280) -> (hi(x)=w270:u8, lo(x)=w269:u8)
            n279 = Split Number(x=w276) -> (hi(x)=w265:u8, lo(x)=w264:u8)
            n280 = Split Number(x=w279) -> (hi(x)=w268:u8, lo(x)=w267:u8)
            n281 = Split Number(x=w275) -> (hi(x)=w263:u8, lo(x)=w262:u8)
            n282 = Split Number(x=w274) -> (hi(x)=w261:u8, lo(x)=w260:u8)
            n283 = Multiply(x=w240, y="Phase count adjustment (DIO)") -> (x*y=w236:i16)
            n284 = feedback #18(i16 0) -> (w238:i16)
            n285 = Subtract(x=w238, y=w236) -> (x-y=w237:i16)
            "DIO Relative phase" <- w237
            n286 = feedback-in #18(w237) -> ()
            n287 = Add(x=w243, y=w236) -> (x+y=w242:u16)
            n288 = Build Array "BD 1 A Stack"(w235, w234) -> (w257:u8[])
            n289 = Build Array "BD 2 A Stack"(w232, w231) -> (w256:u8[])
            n290 = Build Array "BD 1 nu Stack"(w272, w271, w270, w269, w268, w267) -> (w266:u8[])
            n291 = Build Array "BD 2 nu Stack"(w265, w264, w263, w262, w261, w260) -> (w259:u8[])
            n292 = case shown="2" w214 {
              tunnel: [w327 w330] -> w255
              tunnel: [u8 10 u8 4] -> w258
              tunnel: "Swap F1 and F2" -> [w328 w330]
              frame 2 {
                # "F2"
                n293 = Not(x=w328) -> (.not. x?=w327:bool)
              }
              frame 1, Default {
                # "low chooses F1"
                # "F1"
              }
            }
            n294 = case "If FPGA is controlling (toggling) RF synth" shown="True" w254 {
              tunnel: w266 -> [_ w303]
              tunnel: w259 -> [_ w302]
              tunnel: w258 -> [_ w301]
              tunnel: w257 -> [_ w300]
              tunnel: w256 -> [_ w299]
              frame False {
              }
              frame True {
                # "Write next amp.\n(wait until beginning of next loop iteration to update)"
                n295 = flat-sequence "Update the next F1 and F2 frequency value (the actual frequency won't change until FSK is switched).\nThen load the next amplitude value into buffer, but don't update it until the next cycle." {
                  tunnel: w302 -> [w305]
                  tunnel: w303 -> [w306]
                  tunnel: [w306] -> w298
                  tunnel: [w305] -> w297
                  tunnel: w301 -> [w307]
                  tunnel: w298 -> [w309]
                  tunnel: w297 -> [w308]
                  tunnel: w300 -> [w320]
                  tunnel: w299 -> [w319]
                  frame #0 {
                    # "To possibly send\nthese writes to very\nend of loop (for x and\ny phase adjust)"
                    n296 = call "Wait8"("Count(Ticks)"="Next trap write delay (ticks)") -> ()  [unwired: 1 out]
                  }
                  frame #1 {
                    n297 = for {
                      tunnel: w309 -> [w315] mode=indexing
                      tunnel: w308 -> [w314] mode=indexing
                      tunnel: w307 -> [w312]
                      i -> [w313]
                      # "Write next freq."
                      n298 = To Unsigned Byte Integer(number=w313) -> (unsigned 8bit integer=w310:u8)
                      n299 = Add(x=w312, y=w310) -> (x+y=w311:u8)
                      n300 = call "write to RF synth bd.vi"("Address Byte"=w311, "BD 2 Byte"=w314, "BD 1 Byte"=w315) -> ()
                    }
                  }
                  frame #2 {
                    w316 = TRUE ("Connector1/DIO15")
                    # "send udclk high\n(BD 1 and 2)"
                    n301 = xnode "FPGA I/O Node"("Connector1/DIO30"=w316, "Connector1/DIO29"=w316) -> ()  [unwired: 2 in, 2 out]
                  }
                  frame #3 {
                    w317 = FALSE ("Connector1/DIO15")
                    n302 = xnode "FPGA I/O Node"("Connector1/DIO30"=w317, "Connector1/DIO29"=w317) -> ()  [unwired: 2 in, 2 out]
                  }
                  frame #4 {
                    n303 = for {
                      tunnel: w320 -> [w326] mode=indexing
                      tunnel: w319 -> [w325] mode=indexing
                      tunnel: u8 33 -> [w323]
                      i -> [w324]
                      n304 = To Unsigned Byte Integer(number=w324) -> (unsigned 8bit integer=w321:u8)
                      n305 = Add(x=w323, y=w321) -> (x+y=w322:u8)
                      n306 = call "write to RF synth bd.vi"("Address Byte"=w322, "BD 2 Byte"=w325, "BD 1 Byte"=w326) -> ()
                    }
                  }
                }
              }
            }
          }
        }
      }
    }
  }
  n307 = while "APD 1 Counter" {
    tunnel: w4 -> [_]
    stop <- FALSE stop-if-true
    n308 = flat-sequence {
      frame #0 {
        n309 = xnode "FPGA I/O Method Node"("FPGA I/O In"=refnum<k21> "Connector0/DIO0" ("APD 1 DO"), "Timeout"=-1) -> ()  [unwired: 2 out]
      }
      frame #1 {
        n310 = local read "APD1 int gate"() -> (w646:bool)
        n311 = case shown="True" w646 {
          frame False {
          }
          frame True {
            n312 = local read "APD1 out state"() -> (w647:bool)
            n313 = case shown="True" w647 {
              frame False {
                n314 = local read "APD 1 Counts 0"() -> (w649:u32)
                n315 = Increment(x=w649) -> (x+1=→"APD 1 Counts 0":u32)
              }
              frame True {
                n316 = local read "APD 1 Counts 1"() -> (w651:u32)
                n317 = Increment(x=w651) -> (x+1=→"APD 1 Counts 1":u32)
              }
            }
          }
        }
      }
    }
  }
  n318 = while "APD 2 Counter" {
    tunnel: w4 -> [_]
    stop <- FALSE stop-if-true
    n319 = flat-sequence {
      frame #0 {
        n320 = xnode "FPGA I/O Method Node"("FPGA I/O In"=refnum<k21> "Connector0/DIO1" ("APD 2 DO"), "Timeout"=-1) -> ()  [unwired: 2 out]
      }
      frame #1 {
        n321 = local read "APD2 int gate"() -> (w655:bool)
        n322 = case shown="True" w655 {
          frame False {
          }
          frame True {
            n323 = local read "APD2 out state"() -> (w656:bool)
            n324 = case shown="False" w656 {
              frame False {
                n325 = local read "APD 2 Counts 0"() -> (w658:u32)
                n326 = Increment(x=w658) -> (x+1=→"APD 2 Counts 0":u32)
              }
              frame True {
                n327 = local read "APD 2 Counts 1"() -> (w660:u32)
                n328 = Increment(x=w660) -> (x+1=→"APD 2 Counts 1":u32)
              }
            }
          }
        }
      }
    }
  }
  n329 = while "APD 2 Gating" {
    shift-right: [w664] -> _
    shift-left: w4 -> [w669]
    shift-right: [w663] -> _
    shift-left: w7 -> [w661]
    stop <- FALSE stop-if-true
    n330 = flat-sequence {
      tunnel: w669 -> [w672]
      tunnel: [w673] -> w667
      tunnel: [w672] -> w665
      tunnel: [w671] -> w662
      tunnel: w661 -> [w671]
      tunnel: [w676] -> w668
      tunnel: w667 -> [w676]
      tunnel: [w675] -> w666
      tunnel: w665 -> [w675]
      tunnel: w662 -> [w674]
      tunnel: [w698] -> w664
      tunnel: w668 -> [w708]
      tunnel: w666 -> [w706]
      tunnel: [w677] -> w663
      frame #0 {
        n331 = call "Loop Timer8"("Count(Ticks)"=w672) -> ("Tick Count(Ticks)"=w673:u16)
      }
      frame #1 {
        # "Signal maybe then sent through \na transistor before APD"
        n332 = xnode "FPGA I/O Node"("Connector0/DIO8"=w674, "Connector0/DIO9"=w674, "Connector0/DIO10"=w674, "Connector0/DIO11"=w674) -> ()  [unwired: 4 in, 4 out]
        "APD2 int gate" <- w674
      }
      frame #2 {
        n333 = local read "APD Gate ON Count"() -> (w691:u16)
        n334 = local read "APD Gate OFF Count"() -> (w690:u16)
        n335 = feedback #19(TRUE) -> (w703:bool)
        n336 = feedback-in #20(w708) -> ()
        n337 = feedback #20(w708) -> (w692:u16)
        n338 = Not(x=w703) -> (.not. x?=w701:bool)
        n339 = feedback-in #19(w701) -> ()
        n340 = Subtract(x=w708, y=w692) -> (x-y=w707:u16)
        n341 = Select(t=w691, s=w701, f=w690) -> (s? t:f=w705:u16)
        n342 = Subtract(x=w707, y=w706) -> (x-y=w683:u16)
        n343 = Subtract(x=w705, y=w683) -> (x-y=w697:u16)
        n344 = Number To Boolean Array(number=w683) -> (Boolean array=w682:bool[])
        n345 = Or Array Elements(Boolean array=w682) -> (logical OR=w681:bool)
        n346 = Boolean To (0,1)(Boolean="+ phase (APD 2 Gate)") -> (0, 1=w695:i16)
        n347 = Multiply(x=w695, y="Phase count adjustment (APD 2 Gate)") -> (x*y=w693:i16)
        n348 = Boolean To (0,1)(Boolean=w681) -> (0, 1=w688:i16)
        n349 = Add(x=w697, y=w693) -> (x+y=w698:u16)
        n350 = To Unsigned Byte Integer(number=w688) -> (unsigned 8bit integer=w685:u8)
        n351 = feedback #21(i16 0) -> (w700:i16)
        n352 = Subtract(x=w700, y=w693) -> (x-y=w699:i16)
        "APD 2 Gate Relative Phase" <- w699
        n353 = feedback-in #21(w699) -> ()
        n354 = feedback #22(u8 0) -> (w686:u8)
        n355 = Add(x=w685, y=w686) -> (x+y=w684:u8)
        "APD 2 Gate Late Counter" <- w684
        n356 = feedback-in #22(w684) -> ()
        n357 = local read "APD Gate Operating Mode"() -> (w689:u8)
        n358 = case shown="2" w689 {
          tunnel: [TRUE FALSE w711] -> w678
          tunnel: w703 -> [_ _ w711]
          frame 0, Default {
          }
          frame 1 {
          }
          frame 2 {
          }
        }
        n359 = local read "Invert APD Gate"() -> (w680:bool)
        n360 = Not(x=w678) -> (.not. x?=w679:bool)
        n361 = Select(t=w679, s=w680, f=w678) -> (s? t:f=w677:bool)
      }
    }
  }
  n362 = while "532 nm green fluorescent laser interlacing (DO to IA 532 nm AOM ME amp)." {
    shift-right: [w715] -> _
    shift-left: w4 -> [w720]
    shift-right: [w714] -> _
    shift-left: w5 -> [w712]
    stop <- FALSE stop-if-true
    n363 = flat-sequence {
      tunnel: w720 -> [w723]
      tunnel: [w724] -> w718
      tunnel: [w723] -> w716
      tunnel: [w722] -> w713
      tunnel: w712 -> [w722]
      tunnel: [w727] -> w719
      tunnel: w718 -> [w727]
      tunnel: [w726] -> w717
      tunnel: w716 -> [w726]
      tunnel: w713 -> [w725]
      tunnel: [w736] -> w715
      tunnel: w719 -> [w756]
      tunnel: w717 -> [w753]
      tunnel: [w745] -> w714
      frame #0 {
        n364 = call "Loop Timer4"("Count(Ticks)"=w723) -> ("Tick Count(Ticks)"=w724:u16)
      }
      frame #1 {
        n365 = xnode "FPGA I/O Node"("Connector1/DIO34"=w725, "Connector1/DIO38"=w725, "Connector1/DIO39"=w725) -> ()  [unwired: 3 in, 3 out]
      }
      frame #2 {
        n366 = feedback-in #23(w756) -> ()
        n367 = feedback #23(w756) -> (w755:u16)
        n368 = Subtract(x=w756, y=w755) -> (x-y=w754:u16)
        n369 = Subtract(x=w754, y=w753) -> (x-y=w729:u16)
        n370 = Number To Boolean Array(number=w729) -> (Boolean array=w730:bool[])
        n371 = Or Array Elements(Boolean array=w730) -> (logical OR=w728:bool)
        n372 = Boolean To (0,1)(Boolean="+ phase (GI)") -> (0, 1=w741:i16)
        n373 = Multiply(x=w741, y="Phase count adjustment (GI)") -> (x*y=w738:i16)
        n374 = Boolean To (0,1)(Boolean=w728) -> (0, 1=w735:i16)
        n375 = To Unsigned Byte Integer(number=w735) -> (unsigned 8bit integer=w732:u8)
        n376 = feedback #24(i16 0) -> (w739:i16)
        n377 = feedback #25(u8 0) -> (w733:u8)
        n378 = Add(x=w732, y=w733) -> (x+y=w731:u8)
        "GI Late Counter" <- w731
        n379 = feedback-in #25(w731) -> ()
        n380 = Subtract(x=w739, y=w738) -> (x-y=w737:i16)
        "GI Relative phase" <- w737
        n381 = feedback-in #24(w737) -> ()
        n382 = feedback #26(TRUE) -> (w748:bool)
        n383 = case shown="2" "Operating Mode" {
          tunnel: [TRUE FALSE w762] -> w745
          tunnel: w748 -> [_ _ w759]
          frame 0, Default {
          }
          frame 1 {
          }
          frame 2 {
            n384 = Not(x=w759) -> (.not. x?=w761:bool)
            n385 = Select(t=w761, s="Invert GI", f=w759) -> (s? t:f=w762:bool)
          }
        }
        n386 = Not(x=w748) -> (.not. x?=w744:bool)
        n387 = Select(t="Green interlace ON count", s=w744, f="Green interlace OFF count") -> (s? t:f=w750:u16)
        n388 = Subtract(x=w750, y=w729) -> (x-y=w742:u16)
        n389 = Add(x=w742, y=w738) -> (x+y=w736:u16)
        n390 = feedback-in #26(w744) -> ()
      }
    }
  }
  n391 = while "Green and red fluorescent laser interlacing (Current AO to IA 532 nm AOM ME amp)." {
    shift-right: [w771] -> _
    shift-left: w4 -> [w774]
    shift-right: [w768] -> _
    shift-left: w6 -> [w766]
    shift-right: [w765] -> _
    shift-left: w6 -> [w764]
    stop <- FALSE stop-if-true
    n392 = flat-sequence {
      tunnel: w774 -> [w778]
      tunnel: [w779] -> w773
      tunnel: [w778] -> w772
      tunnel: [w777] -> w767
      tunnel: w766 -> [w777]
      tunnel: w764 -> [w776]
      tunnel: [w776] -> w763
      tunnel: [w783] -> w770
      tunnel: w773 -> [w783]
      tunnel: [w782] -> w769
      tunnel: w772 -> [w782]
      tunnel: w767 -> [w781]
      tunnel: w763 -> [w780]
      tunnel: [w796] -> w771
      tunnel: [w812] -> w768
      tunnel: w770 -> [w823]
      tunnel: w769 -> [w820]
      tunnel: [w786] -> w765
      frame #0 {
        n393 = call "Loop Timer10"("Count(Ticks)"=w778) -> ("Tick Count(Ticks)"=w779:u16)
      }
      frame #1 {
        n394 = xnode "FPGA I/O Node"("Chassis2/Mod1/AO0"=w781, "Chassis2/Mod1/AO1"=w780) -> ()  [unwired: 2 in, 2 out]
      }
      frame #2 {
        # "Design note:\n\nThese two laser controls are in the same loop\nbecause the expansion current AI cannot separately\ntime the outputs fast enough for us.  Apparently\nit is because of communication time between the\nexpansion card and the fpga.\n\nSo the two analog control signals have the same timing\nand profile, but independent amplitudes to independently\ncontrol the intensity and feedback for each laser."
        n395 = feedback #27(TRUE) -> (w784:bool)
        n396 = Not(x=w784) -> (.not. x?=w785:bool)
        n397 = feedback-in #27(w785) -> ()
        n398 = Subtract(x="Green interlace OFF count 2", y="Green int current ON count adj") -> (x-y=w805:u16)
        n399 = disable-structure shown="Disabled" {
          disable-tunnel: [w827 _] -> w786
          disable-tunnel: w784 -> [w824 _]
          frame Disabled {
            n400 = case shown="2" "RI Operating Mode 2" {
              tunnel: [TRUE FALSE w839] -> w825
              tunnel: w824 -> [_ _ w836]
              frame 0, Default {
              }
              frame 1 {
              }
              frame 2 {
                n401 = Not(x=w836) -> (.not. x?=w838:bool)
                n402 = Select(t=w838, s="Invert RI 2", f=w836) -> (s? t:f=w839:bool)
              }
            }
            n403 = And(x=w825, y="Red FB On/Off") -> (x .and. y?=w833:bool)
            n404 = case shown="True" w833 {
              tunnel: "RI Current Out" -> [w840 _]
              tunnel: [w840 w849] -> w829
              frame False {
              }
              frame True {
                n405 = local read "Red FB Intensity"() -> (w845:i16)
                n406 = Bundle("P4"="P4", "I4"="I4", "D4"="D4") -> (w841:cluster{"P4":i16, "I4":i16, "D4":i16})  [unwired: 1 in]
                n407 = call "Slower PID.vi"("process variable"=w845, "reset?"="Red FB Reset", "setpoint"="Red FB Setpoint", "PID gains (x 2^8)"=w841, "output range"=cluster{"output high":i16, "output low":i16} {"output high"=32767, "output low"=-32768} ("Green FB output range")) -> ("output"=w852:i16)  [unwired: 10 out]
                n408 = To Long Integer(number=w852) -> (32bit integer=w846:i32)
                n409 = Add(x=w846, y=32768) -> (x+y=w848:i32)
                n410 = To Unsigned Word Integer(number=w848) -> (unsigned 16bit integer=w849:u16)
              }
            }
            n411 = Boolean To (0,1)(Boolean=w825) -> (0, 1=w828:i16)
            n412 = To Unsigned Word Integer(number=w828) -> (unsigned 16bit integer=w830:u16)
            n413 = Multiply(x=w830, y=w829) -> (x*y=w827:u16)
          }
          frame Enabled {
          }
        }
        n414 = feedback-in #28(w823) -> ()
        n415 = feedback #28(w823) -> (w822:u16)
        n416 = Add(x="Green int current ON count adj", y="Green interlace ON count 2") -> (x+y=w806:u16)
        n417 = Subtract(x=w823, y=w822) -> (x-y=w821:u16)
        n418 = Select(t=w806, s=w785, f=w805) -> (s? t:f=w817:u16)
        n419 = Subtract(x=w821, y=w820) -> (x-y=w789:u16)
        n420 = Subtract(x=w817, y=w789) -> (x-y=w800:u16)
        n421 = case shown="2" "Operating Mode 2" {
          tunnel: [TRUE FALSE w873] -> w787
          tunnel: w784 -> [_ _ w870]
          frame 0, Default {
          }
          frame 1 {
          }
          frame 2 {
            n422 = Not(x=w870) -> (.not. x?=w872:bool)
            n423 = Select(t=w872, s="Invert GI 2", f=w870) -> (s? t:f=w873:bool)
          }
        }
        n424 = Number To Boolean Array(number=w789) -> (Boolean array=w790:bool[])
        n425 = Boolean To (0,1)(Boolean="+ phase (GI) 2") -> (0, 1=w802:i16)
        n426 = Or Array Elements(Boolean array=w790) -> (logical OR=w788:bool)
        n427 = Boolean To (0,1)(Boolean=w788) -> (0, 1=w795:i16)
        n428 = Multiply(x=w802, y="Phase count adjustment (GI) 2") -> (x*y=w798:i16)
        n429 = To Unsigned Byte Integer(number=w795) -> (unsigned 8bit integer=w791:u8)
        n430 = Add(x=w800, y=w798) -> (x+y=w796:u16)
        n431 = feedback #29(u8 0) -> (w793:u8)
        n432 = Add(x=w791, y=w793) -> (x+y=w792:u8)
        "GI Late Counter 2" <- w792
        n433 = feedback-in #29(w792) -> ()
        n434 = feedback #30(i16 0) -> (w799:i16)
        n435 = Subtract(x=w799, y=w798) -> (x-y=w797:i16)
        "GI Relative phase 2" <- w797
        n436 = feedback-in #30(w797) -> ()
        n437 = And(x=w787, y="Green FB On/Off") -> (x .and. y?=w807:bool)
        n438 = case shown="False" w807 {
          tunnel: "Current Out" -> [w854 _]
          tunnel: [w854 w863] -> w811
          frame False {
          }
          frame True {
            n439 = local read "Green FB Sum"() -> (w859:i16)
            n440 = Bundle("P3"="P3", "I3"="I3", "D3"="D3") -> (w855:cluster{"P3":i16, "I3":i16, "D3":i16})  [unwired: 1 in]
            n441 = call "Slower PID.vi"("process variable"=w859, "reset?"="Green FB Reset", "setpoint"="Green FB Setpoint", "PID gains (x 2^8)"=w855, "output range"=cluster{"output high":i16, "output low":i16} {"output high"=32767, "output low"=-32768} ("Green FB output range")) -> ("output"=w866:i16)  [unwired: 10 out]
            n442 = To Long Integer(number=w866) -> (32bit integer=w860:i32)
            n443 = Add(x=w860, y=32768) -> (x+y=w862:i32)
            n444 = To Unsigned Word Integer(number=w862) -> (unsigned 16bit integer=w863:u16)
          }
        }
        n445 = Boolean To (0,1)(Boolean=w787) -> (0, 1=w813:i16)
        n446 = To Unsigned Word Integer(number=w813) -> (unsigned 16bit integer=w810:u16)
        n447 = Multiply(x=w810, y=w811) -> (x*y=w812:u16)
      }
    }
  }
  n448 = while "APD 1 Gating" {
    shift-right: [w877] -> _
    shift-left: w4 -> [w882]
    shift-right: [w876] -> _
    shift-left: w7 -> [w874]
    stop <- FALSE stop-if-true
    n449 = flat-sequence {
      tunnel: w882 -> [w885]
      tunnel: [w886] -> w880
      tunnel: [w885] -> w878
      tunnel: [w884] -> w875
      tunnel: w874 -> [w884]
      tunnel: [w889] -> w881
      tunnel: w880 -> [w889]
      tunnel: [w888] -> w879
      tunnel: w878 -> [w888]
      tunnel: w875 -> [w887]
      tunnel: [w907] -> w877
      tunnel: w881 -> [w921]
      tunnel: w879 -> [w918]
      tunnel: [w890] -> w876
      frame #0 {
        n450 = call "Loop Timer7"("Count(Ticks)"=w885) -> ("Tick Count(Ticks)"=w886:u16)
      }
      frame #1 {
        # "Signal maybe then sent through \na transistor before APD"
        n451 = xnode "FPGA I/O Node"("Connector0/DIO4"=w887, "Connector0/DIO5"=w887, "Connector0/DIO6"=w887, "Connector0/DIO7"=w887) -> ()  [unwired: 4 in, 4 out]
        "APD1 int gate" <- w887
      }
      frame #2 {
        n452 = feedback #31(TRUE) -> (w913:bool)
        n453 = feedback-in #32(w921) -> ()
        n454 = feedback #32(w921) -> (w920:u16)
        n455 = Not(x=w913) -> (.not. x?=w910:bool)
        n456 = feedback-in #31(w910) -> ()
        n457 = Subtract(x=w921, y=w920) -> (x-y=w919:u16)
        n458 = Select(t="APD Gate ON Count", s=w910, f="APD Gate OFF Count") -> (s? t:f=w915:u16)
        n459 = Subtract(x=w919, y=w918) -> (x-y=w895:u16)
        n460 = Subtract(x=w915, y=w895) -> (x-y=w906:u16)
        n461 = Number To Boolean Array(number=w895) -> (Boolean array=w896:bool[])
        n462 = Or Array Elements(Boolean array=w896) -> (logical OR=w894:bool)
        n463 = Boolean To (0,1)(Boolean="+ phase (APD 1 Gate)") -> (0, 1=w904:i16)
        n464 = Boolean To (0,1)(Boolean=w894) -> (0, 1=w901:i16)
        n465 = Multiply(x=w904, y="Phase count adjustment (APD 1 Gate)") -> (x*y=w902:i16)
        n466 = To Unsigned Byte Integer(number=w901) -> (unsigned 8bit integer=w898:u8)
        n467 = Add(x=w906, y=w902) -> (x+y=w907:u16)
        n468 = feedback #33(i16 0) -> (w909:i16)
        n469 = Subtract(x=w909, y=w902) -> (x-y=w908:i16)
        "APD 1 Gate Relative Phase" <- w908
        n470 = feedback-in #33(w908) -> ()
        n471 = feedback #34(u8 0) -> (w899:u8)
        n472 = Add(x=w898, y=w899) -> (x+y=w897:u8)
        "APD 1 Gate Late Counter" <- w897
        n473 = feedback-in #34(w897) -> ()
        n474 = case shown="2" "APD Gate Operating Mode" {
          tunnel: [TRUE FALSE w924] -> w891
          tunnel: w913 -> [_ _ w924]
          frame 0, Default {
          }
          frame 1 {
          }
          frame 2 {
          }
        }
        n475 = Not(x=w891) -> (.not. x?=w892:bool)
        n476 = Select(t=w892, s="Invert APD Gate", f=w891) -> (s? t:f=w890:bool)
      }
    }
  }
  n477 = while "MCL stage control" {
    shift-right: [w937] -> _
    shift-left: w4 -> [w940]
    shift-right: [w930] -> _
    shift-left: w12 -> [w927]
    shift-right: [w929] -> _
    shift-left: w11 -> [w925]
    stop <- FALSE stop-if-true
    n478 = flat-sequence {
      tunnel: w940 -> [w944]
      tunnel: [w945] -> w936
      tunnel: [w944] -> w934
      tunnel: [w943] -> w928
      tunnel: w927 -> [w943]
      tunnel: [w942] -> w926
      tunnel: w925 -> [w942]
      tunnel: w936 -> [w949]
      tunnel: [w949] -> w935
      tunnel: w934 -> [w948]
      tunnel: [w948] -> w933
      tunnel: w928 -> [w947]
      tunnel: w926 -> [w946]
      tunnel: w935 -> [w957]
      tunnel: w933 -> [w956]
      tunnel: [w957] -> w939
      tunnel: [w956] -> w938
      tunnel: [w955] -> w932
      tunnel: [w954] -> w931
      tunnel: [w1029] -> w937
      tunnel: w939 -> [w1036]
      tunnel: w938 -> [w1033]
      tunnel: w932 -> [w1031]
      tunnel: w931 -> [w1030]
      tunnel: [w1031] -> w930
      tunnel: [w1030] -> w929
      frame #0 {
        n479 = call "Loop Timer5"("Count(Ticks)"=w944) -> ("Tick Count(Ticks)"=w945:u32)
      }
      frame #1 {
        n480 = xnode "FPGA I/O Node"("Connector0/AO1"=w947, "Connector0/AO2"=w946) -> ()  [unwired: 2 in, 2 out]
      }
      frame #2 {
        n481 = local read "Scanning MCL"() -> (w969:bool)
        n482 = Or(x=w969, y="Start scan (MCL)") -> (x .or. y?=w964:bool)
        n483 = Not(x="Abort scan (MCL)") -> (.not. x?=w962:bool)
        n484 = And(x=w962, y=w964) -> (x .and. y?=w961:bool)
        n485 = case "Raster scan" shown="True" w961 {
          tunnel: [w970 w1013] -> w966
          tunnel: "Start scan (MCL)" -> [_ w998]
          tunnel: [w970 w974] -> w950
          frame False {
            w970 = i16 0
            n486 = local write "Scanning MCL"(FALSE ("scanning")) -> ()
          }
          frame True {
            w984 = i16 0
            w983 = u64 0
            # "scan incr."
            # "freq. incr. mult."
            # "count steps"
            # "count number of cycles"
            n487 = feedback #35(w983) -> (w1010:u64)
            n488 = Select(t=w983, s=w998, f=w1010) -> (s? t:f=w1012:u64)
            n489 = Increment(x=w1012) -> (x+1=w1009:u64)
            n490 = Greater?(x="Cycles per step (MCL)", y=w1009) -> (0:w993:bool)
            n491 = Select(t=w1009, s=w993, f=w983) -> (s? t:f=w1008:u64)
            n492 = feedback-in #35(w1008) -> ()
            n493 = feedback #36(w983) -> (w1007:u64)
            n494 = Select(t=w983, s=w998, f=w1007) -> (s? t:f=w1002:u64)
            n495 = Increment(x=w1002) -> (x+1=w1006:u64)
            n496 = Add(x="Scan steps (MCL)", y="Scan steps (MCL)") -> (x+y=w1005:u64)
            n497 = Select(t=w1002, s=w993, f=w1006) -> (s? t:f=w988:u64)
            n498 = Greater?(x=w1005, y=w988) -> (0:w987:bool)
            n499 = Select(t=w988, s=w987, f=w983) -> (s? t:f=w1003:u64)
            n500 = feedback-in #36(w1003) -> ()
            n501 = Equal?(x="Scan steps (MCL)", y=w988) -> (x = y?=w992:bool)
            n502 = Greater?(x="Scan steps (MCL)", y=w1002) -> (0:w1001:bool)
            n503 = feedback #37(w984) -> (w1004:i16)
            n504 = Select(t=w984, s=w998, f=w1004) -> (s? t:f=w990:i16)
            n505 = Increment(x=w990) -> (x+1=w1000:i16)
            n506 = Decrement(x=w990) -> (x-1=w999:i16)
            n507 = Select(t=w1000, s=w1001, f=w999) -> (s? t:f=w991:i16)
            n508 = Select(t=w990, s=w992, f=w991) -> (s? t:f=w989:i16)
            n509 = Select(t=w990, s=w993, f=w989) -> (s? t:f=w985:i16)
            n510 = Select(t=w985, s=w987, f=w984) -> (s? t:f=w986:i16)
            n511 = feedback-in #37(w986) -> ()
            n512 = feedback #38(w983) -> (w997:u64)
            n513 = Select(t=w983, s=w998, f=w997) -> (s? t:f=w972:u64)
            n514 = Increment(x=w972) -> (x+1=w994:u64)
            n515 = Select(t=w972, s=w987, f=w994) -> (s? t:f=w973:u64)
            n516 = Greater?(x="Number of scans (MCL)", y=w973) -> (0:w980:bool)
            n517 = Multiply(x="Scan freq.  increment (MCL)", y=w990) -> (x*y=w1013:i16)
            n518 = Select(t=TRUE, s="Cont. Scan (MCL)", f=w980) -> (s? t:f=w979:bool)
            "Scanning MCL" <- w979
            n519 = Select(t=w973, s=w979, f=w983) -> (s? t:f=w995:u64)
            n520 = feedback-in #38(w995) -> ()
            n521 = Increment(x=w973) -> (x+1=→"Scan I (MCL)":u64)
            n522 = To Word Integer(number=w972) -> (16bit integer=w975:i16)
            n523 = Multiply(x=w975, y="Scan freq.  increment (MCL)") -> (x*y=w974:i16)
          }
        }
        n524 = Select(t=w950, s="1D or 2D Scan?", f=i16 0) -> (s? t:f=w951:i16)
        n525 = Select(t=w951, s="MCL Scan Axis", f=w966) -> (s? t:f=w965:i16)
        n526 = Select(t=w966, s="MCL Scan Axis", f=w951) -> (s? t:f=w967:i16)
        n527 = Add(x=w965, y="AO2") -> (x+y=w954:i16)
        n528 = Add(x="AO1", y=w967) -> (x+y=w955:i16)
      }
      frame #3 {
        n529 = feedback-in #39(w1036) -> ()
        n530 = feedback #39(w1036) -> (w1035:u32)
        n531 = Boolean To (0,1)(Boolean="+ phase (MCL)") -> (0, 1=w1027:i16)
        n532 = Subtract(x=w1036, y=w1035) -> (x-y=w1034:u32)
        n533 = Multiply(x=w1027, y="Phase count adjustment (MCL)") -> (x*y=w1023:i16)
        n534 = Subtract(x=w1034, y=w1033) -> (x-y=w1015:u32)
        n535 = Subtract(x="MCL count", y=w1015) -> (x-y=w1025:u32)
        n536 = feedback #40(i16 0) -> (w1024:i16)
        n537 = Subtract(x=w1024, y=w1023) -> (x-y=w1022:i16)
        "MCL Relative Phase" <- w1022
        n538 = feedback-in #40(w1022) -> ()
        n539 = Number To Boolean Array(number=w1015) -> (Boolean array=w1016:bool[])
        n540 = Or Array Elements(Boolean array=w1016) -> (logical OR=w1014:bool)
        n541 = Boolean To (0,1)(Boolean=w1014) -> (0, 1=w1021:i16)
        n542 = Add(x=w1025, y=w1023) -> (x+y=w1029:u32)
        n543 = To Unsigned Byte Integer(number=w1021) -> (unsigned 8bit integer=w1018:u8)
        n544 = feedback #41(u8 0) -> (w1019:u8)
        n545 = Add(x=w1018, y=w1019) -> (x+y=w1017:u8)
        "MCL Late Counter" <- w1017
        n546 = feedback-in #41(w1017) -> ()
      }
    }
  }
  n547 = while "Control APD data integration - stream to host" {
    shift-right: [w1041] -> _
    shift-left: w8 -> [w1046]
    stop <- FALSE stop-if-true
    n548 = flat-sequence {
      tunnel: w1046 -> [w1048]
      tunnel: [w1049] -> w1044
      tunnel: [w1048] -> w1042
      tunnel: [w1059] -> w1045
      tunnel: w1044 -> [w1059]
      tunnel: [w1058] -> w1043
      tunnel: w1042 -> [w1058]
      tunnel: [w1057] -> w1040
      tunnel: [w1056] -> w1039
      tunnel: [w1050] -> w1038
      tunnel: [w1101] -> w1041
      tunnel: w1045 -> [w1111]
      tunnel: w1043 -> [w1108]
      tunnel: w1040 -> [w1094]
      tunnel: w1039 -> [w1093]
      tunnel: w1038 -> [w1081]
      frame #0 {
        n549 = call "Loop Timer6"("Count(Ticks)"=w1048) -> ("Tick Count(Ticks)"=w1049:u32)
      }
      frame #1 {
        n550 = flat-sequence {
          tunnel: [w1061] -> w1055
          tunnel: w1055 -> [w1064]
          tunnel: [w1068] -> w1054
          tunnel: [w1067] -> w1053
          tunnel: [w1064] -> w1052
          tunnel: [w1063] -> w1051
          tunnel: [w1075] -> w1056
          tunnel: [w1076] -> w1057
          tunnel: w1054 -> [w1076]
          tunnel: w1053 -> [w1075]
          tunnel: w1052 -> [w1074]
          tunnel: w1051 -> [w1073]
          tunnel: [w1073] -> w1050
          frame #0 {
            # "use separate variable so each APD won't\nhave to wait to read"
            n551 = feedback #42(FALSE) -> (w1060:bool)
            "APD1 out state" <- w1060
            "APD2 out state" <- w1060
            "APD3 out state" <- w1060
            n552 = Not(x=w1060) -> (.not. x?=w1061:bool)
            n553 = feedback-in #42(w1061) -> ()
          }
          frame #1 {
            n554 = local read "APD 3 Counts 1"() -> (w1066:u32)
            n555 = local read "APD 3 Counts 0"() -> (w1065:u32)
            n556 = local read "APD 1 Counts 1"() -> (w1072:u32)
            n557 = local read "APD 1 Counts 0"() -> (w1071:u32)
            n558 = local read "APD 2 Counts 1"() -> (w1070:u32)
            n559 = local read "APD 2 Counts 0"() -> (w1069:u32)
            n560 = Select(t=w1066, s=w1064, f=w1065) -> (s? t:f=w1063:u32)
            n561 = Select(t=w1072, s=w1064, f=w1071) -> (s? t:f=w1068:u32)
            n562 = Select(t=w1070, s=w1064, f=w1069) -> (s? t:f=w1067:u32)
          }
          frame #2 {
            n563 = case shown="False" w1074 {
              frame False {
                w1077 = u32 0 ("APD 1 Counts 0")
                n564 = local write "APD 1 Counts 0"(w1077) -> ()
                n565 = local write "APD 2 Counts 0"(w1077) -> ()
                n566 = local write "APD 3 Counts 0"(w1077) -> ()
              }
              frame True {
                w1078 = u32 0 ("APD 1 Counts 1")
                n567 = local write "APD 1 Counts 1"(w1078) -> ()
                n568 = local write "APD 2 Counts 1"(w1078) -> ()
                n569 = local write "APD 3 Counts 1"(w1078) -> ()
              }
            }
          }
        }
      }
      frame #2 {
        n570 = feedback-in #43(w1111) -> ()
        n571 = feedback #43(w1111) -> (w1110:u32)
        n572 = Subtract(x=w1111, y=w1110) -> (x-y=w1109:u32)
        n573 = Subtract(x=w1109, y=w1108) -> (x-y=w1086:u32)
        n574 = case shown="True" "APD to FIFO" {
          tunnel: w1094 -> [_ w1116]
          tunnel: w1093 -> [_ w1114]
          tunnel: w1081 -> [_ w1112]
          frame False {
          }
          frame True {
            n575 = flat-sequence {
              tunnel: 0 ("Timeout") -> [w1118]
              tunnel: w1116 -> [w1119]
              tunnel: [w1118] -> w1115
              tunnel: w1115 -> [w1120]
              tunnel: w1114 -> [w1121]
              tunnel: [w1120] -> w1113
              tunnel: w1113 -> [w1123]
              tunnel: w1112 -> [w1122]
              frame #0 {
                n576 = xnode ("FIFO Write")("Element"=w1119, "Timeout"=w1118) -> ()  [unwired: 1 in, 2 out]
              }
              frame #1 {
                n577 = xnode ("FIFO Write")("Element"=w1121, "Timeout"=w1120) -> ()  [unwired: 1 in, 2 out]
              }
              frame #2 {
                n578 = xnode ("FIFO Write")("Element"=w1122, "Timeout"=w1123) -> ()  [unwired: 1 in, 2 out]
              }
            }
          }
        }
        n579 = Subtract(x="APD Acq Rate Count", y=w1086) -> (x-y=w1102:u32)
        n580 = Number To Boolean Array(number=w1086) -> (Boolean array=w1087:bool[])
        n581 = Or Array Elements(Boolean array=w1087) -> (logical OR=w1085:bool)
        n582 = Boolean To (0,1)(Boolean=w1085) -> (0, 1=w1092:i16)
        n583 = To Unsigned Byte Integer(number=w1092) -> (unsigned 8bit integer=w1089:u8)
        n584 = feedback #44(u8 0) -> (w1090:u8)
        n585 = Add(x=w1089, y=w1090) -> (x+y=w1088:u8)
        "APD Acq Late Counter" <- w1088
        n586 = feedback-in #44(w1088) -> ()
        n587 = Boolean To (0,1)(Boolean="+ phase (APD Acq)") -> (0, 1=w1098:i16)
        n588 = Multiply(x=w1098, y="Phase Count Adjustment (APD Acq)") -> (x*y=w1095:i16)
        n589 = Add(x=w1102, y=w1095) -> (x+y=w1101:u32)
        n590 = feedback #45(i16 0) -> (w1100:i16)
        n591 = Subtract(x=w1100, y=w1095) -> (x-y=w1097:i16)
        "APD Acq Relative Phase" <- w1097
        n592 = feedback-in #45(w1097) -> ()
        n593 = To Word Integer(number=w1094) -> (16bit integer=w1103:i16)
        n594 = To Word Integer(number=w1081) -> (16bit integer=w1082:i16)
        n595 = To Word Integer(number=w1093) -> (16bit integer=w1104:i16)
        n596 = Multiply(x="APD AO scale factor", y=w1104) -> (x*y=w1083:i16)
        n597 = Multiply(x="APD AO scale factor", y=w1082) -> (x*y=w1079:i16)
        n598 = Multiply(x="APD AO scale factor", y=w1103) -> (x*y=w1084:i16)
        n599 = xnode "FPGA I/O Node"("Connector0/AO6"=w1084, "Connector0/AO7"=w1083, "Connector0/AO5"=w1079) -> ()  [unwired: 3 in, 3 out]
      }
    }
  }
  n600 = while "DAQ AI set 1" {
    shift-right: [w1124] -> _
    shift-left: w4 -> [w1129]
    stop <- FALSE stop-if-true
    n601 = flat-sequence {
      tunnel: w1129 -> [w1139]
      tunnel: [w1140] -> w1127
      tunnel: [w1139] -> w1126
      tunnel: [w1150] -> w1137
      tunnel: [w1149] -> w1136
      tunnel: [w1148] -> w1135
      tunnel: [w1147] -> w1134
      tunnel: [w1146] -> w1133
      tunnel: [w1145] -> w1132
      tunnel: [w1144] -> w1131
      tunnel: [w1143] -> w1130
      tunnel: [w1142] -> w1128
      tunnel: w1127 -> [w1142]
      tunnel: w1126 -> [w1141]
      tunnel: [w1141] -> w1125
      tunnel: [w1180] -> w1124
      tunnel: w1137 -> [w1206]
      tunnel: w1136 -> [w1172]
      tunnel: w1135 -> [w1173]
      tunnel: w1134 -> [w1152]
      tunnel: w1133 -> [w1196]
      tunnel: w1132 -> [w1195]
      tunnel: w1131 -> [w1194]
      tunnel: w1130 -> [w1193]
      tunnel: w1128 -> [w1190]
      tunnel: w1125 -> [w1187]
      frame #0 {
        n602 = call "Loop Timer3"("Count(Ticks)"=w1139) -> ("Tick Count(Ticks)"=w1140:u16)
      }
      frame #1 {
        n603 = xnode "FPGA I/O Node"("Connector1/DIO31"=TRUE ("Connector1/DIO33")) -> ("Connector0/AI0"=w1150:i16, "Connector0/AI1"=w1149:i16, "Connector0/AI2"=w1148:i16, "Connector0/AI3"=w1147:i16, "Connector0/AI4"=w1146:i16, "Connector0/AI5"=w1145:i16, "Connector0/AI6"=w1144:i16, "Connector0/AI7"=w1143:i16)  [unwired: 9 in, 9 out]
      }
      frame #2 {
        w1176 = FALSE ("AI to FIFO")
        # "Adjust phase after data acquired if button pressed"
        n604 = feedback #46(i16 1) -> (w1199:i16)
        n605 = Increment(x=w1199) -> (x+1=w1205:i16)
        n606 = Scale By Power Of 2(n="AI1 X Scale", x=w1172) -> (x*2^n=w1170:i16)
        n607 = Greater?(x=w1205, y="N of AI1 Int Acq Sets") -> (0:w1202:bool)
        n608 = Select(t=i16 1, s=w1202, f=w1205) -> (s? t:f=w1204:i16)
        n609 = feedback-in #46(w1204) -> ()
        n610 = Divide(x=w1170, y=w1152) -> (x/y=w1169:fxp<+/-,16,1>)
        n611 = feedback #47(w1176) -> (w1174:bool)
        n612 = feedback #48(w1176) -> (w1192:bool)
        n613 = case shown="2" w1199 {
          tunnel: w1173 -> [w1229 w1236 _]
          tunnel: ["Set 1" "Set 2" "Set 3"] -> w1197
          tunnel: ["AI to FIFO" w1238 w1243] -> w1191
          tunnel: w1192 -> [_ w1238 w1243]
          tunnel: ["Trap Pos to FIFO" w1237 w1242] -> w1175
          tunnel: w1174 -> [_ w1237 w1242]
          tunnel: w1169 -> [w1228 w1235 _]
          tunnel: [w1227 w1233 FALSE] -> w1156
          tunnel: [w1226 w1234 u64 0 ("BD1 Frequency Out 2")] -> w1155
          frame 1, Default {
            n614 = local read "BD1 Frequency Out 1"() -> (w1226:u64)
            n615 = Compound Arithmetic op=AND("Trap Pos to FIFO", "Set 1", "AI to FIFO") -> (w1227:bool)
            "AI2 Y Sum Set 1" <- w1229
            "AI1 X Set 1" <- w1228
          }
          frame 2 {
            n616 = local read "BD1 Frequency Out 2"() -> (w1234:u64)
            n617 = Compound Arithmetic op=AND(w1237, "Set 2", w1238) -> (w1233:bool)
            "AI2 Y Sum Set 2" <- w1236
            "AI1 X Set 2" <- w1235
          }
          frame 3 {
          }
        }
        n618 = And(x=w1197, y=w1191) -> (x .and. y?=w1198:bool)
        n619 = case shown="True" w1198 {
          tunnel: w1206 -> [_ w1257]
          tunnel: w1172 -> [_ w1256]
          tunnel: w1173 -> [_ w1255]
          tunnel: w1152 -> [_ w1254]
          tunnel: w1196 -> [_ w1253]
          tunnel: w1195 -> [_ w1252]
          tunnel: w1194 -> [_ w1251]
          tunnel: w1193 -> [_ w1250]
          tunnel: 0 ("DMA buffer timeout") -> [_ w1259]
          frame False {
          }
          frame True {
            n620 = Build Array(w1257, w1256, w1255, w1254, w1253, w1252, w1251, w1250) -> (w1258:i16[])
            n621 = for {
              tunnel: w1258 -> [w1261] mode=indexing
              tunnel: w1259 -> [w1262]
              tunnel: [w1260] -> w1248 mode=indexing
              n622 = xnode ("FIFO Write")("Element"=w1261, "Timeout"=w1262) -> ("Timed Out?"=w1260:bool)  [unwired: 1 in, 1 out]
            }
            n623 = Or Array Elements(Boolean array=w1248) -> (logical OR=w1245:bool)
            n624 = Boolean To (0,1)(Boolean=w1245) -> (0, 1=w1247:i16)
            n625 = feedback #49(u16 0) -> (w1246:u16)
            n626 = Add(x=w1247, y=w1246) -> (x+y=w1244:u16)
            "Trap AI FIFO Timeout" <- w1244
            n627 = feedback-in #49(w1244) -> ()
          }
        }
        n628 = feedback-in #47(w1175) -> ()
        n629 = feedback-in #48(w1191) -> ()
        n630 = case shown="True" w1156 {
          tunnel: w1155 -> [_ w1212]
          tunnel: [u8 0 w1209] -> w1154
          frame False {
          }
          frame True {
            n631 = Split Number(x=w1212) -> (hi(x)=w1213:u32, lo(x)=w1214:u32)
            n632 = Split Number(x=w1213) -> (lo(x)=w1215:u16)  [unwired: 1 out]
            n633 = Split Number(x=w1214) -> (hi(x)=w1216:u16, lo(x)=w1217:u16)
            n634 = Build Array "BD 1 nu Stack"(w1215, w1216, w1217) -> (w1211:u16[])
            n635 = for {
              tunnel: w1211 -> [w1224] mode=indexing
              shift-right: [w1220] -> w1209
              shift-left: u8 0 -> [w1221]
              n636 = xnode ("FIFO Method Node")("Element"=w1224, "Timeout"="Trap FIFO Set Timeout") -> ("Timed Out?"=w1223:bool)  [unwired: 1 in, 1 out]
              n637 = Boolean To (0,1)(Boolean=w1223) -> (0, 1=w1222:i16)
              n638 = To Unsigned Byte Integer(number=w1222) -> (unsigned 8bit integer=w1219:u8)
              n639 = Add(x=w1219, y=w1221) -> (x+y=w1220:u8)
            }
          }
        }
        n640 = To Unsigned Word Integer(number=w1154) -> (unsigned 16bit integer=w1153:u16)
        n641 = feedback #50(u16 0) -> (w1167:u16)
        n642 = Add(x=w1153, y=w1167) -> (x+y=w1166:u16)
        "Trap Pos FIFO Timeout" <- w1166
        n643 = feedback-in #50(w1166) -> ()
        n644 = feedback-in #51(w1190) -> ()
        n645 = feedback #51(w1190) -> (w1189:u16)
        n646 = Subtract(x=w1190, y=w1189) -> (x-y=w1188:u16)
        n647 = xnode "FPGA I/O Node"("Connector1/DIO31"=FALSE ("Connector1/DIO34")) -> ()  [unwired: 1 in, 1 out]
        n648 = Subtract(x=w1188, y=w1187) -> (x-y=w1158:u16)
        n649 = Boolean To (0,1)(Boolean="+ phase") -> (0, 1=w1183:i16)
        n650 = Multiply(x=w1183, y="Phase count adjustment") -> (x*y=w1177:i16)
        n651 = Subtract(x="ai count", y=w1158) -> (x-y=w1181:u16)
        n652 = Number To Boolean Array(number=w1158) -> (Boolean array=w1159:bool[])
        n653 = feedback #52(i16 0) -> (w1179:i16)
        n654 = Add(x=w1181, y=w1177) -> (x+y=w1180:u16)
        n655 = Subtract(x=w1179, y=w1177) -> (x-y=w1178:i16)
        "Relative phase" <- w1178
        n656 = feedback-in #52(w1178) -> ()
        n657 = Or Array Elements(Boolean array=w1159) -> (logical OR=w1157:bool)
        n658 = Boolean To (0,1)(Boolean=w1157) -> (0, 1=w1164:i16)
        n659 = To Unsigned Byte Integer(number=w1164) -> (unsigned 8bit integer=w1161:u8)
        n660 = feedback #53(u8 0) -> (w1162:u8)
        n661 = Add(x=w1161, y=w1162) -> (x+y=w1160:u8)
        "AI Late Counter" <- w1160
        n662 = feedback-in #53(w1160) -> ()
      }
    }
  }
  n663 = node-c288(w9) -> ()
  n664 = disable-structure shown="Disabled" {
    disable-tunnel: w4 -> [w1263 _]
    frame Disabled {
      n665 = while "APD 3 Counter" {
        tunnel: w1263 -> [_]
        stop <- FALSE stop-if-true
        n666 = flat-sequence {
          frame #0 {
            n667 = xnode "FPGA I/O Method Node"("FPGA I/O In"=refnum<k21> "Connector0/DIO2" ("APD 2 DO"), "Timeout"=-1) -> ()  [unwired: 2 out]
          }
          frame #1 {
            n668 = local read "APD3 int gate"() -> (w1267:bool)
            n669 = case shown="True" w1267 {
              frame False {
              }
              frame True {
                n670 = local read "APD3 out state"() -> (w1268:bool)
                n671 = case shown="True" w1268 {
                  frame False {
                    n672 = local read "APD 3 Counts 0"() -> (w1270:u32)
                    n673 = Increment(x=w1270) -> (x+1=→"APD 3 Counts 0":u32)
                  }
                  frame True {
                    n674 = local read "APD 3 Counts 1"() -> (w1272:u32)
                    n675 = Increment(x=w1272) -> (x+1=→"APD 3 Counts 1":u32)
                  }
                }
              }
            }
          }
        }
      }
    }
    frame Enabled {
    }
  }
  n676 = disable-structure shown="Disabled" {
    disable-tunnel: w7 -> [w1274 _]
    disable-tunnel: w4 -> [w1273 _]
    frame Disabled {
      n677 = while "APD 3 Gating" {
        shift-right: [w1278] -> _
        shift-left: w1273 -> [w1283]
        shift-right: [w1277] -> _
        shift-left: w1274 -> [w1275]
        stop <- FALSE stop-if-true
        n678 = flat-sequence {
          tunnel: w1283 -> [w1286]
          tunnel: [w1287] -> w1281
          tunnel: [w1286] -> w1279
          tunnel: [w1285] -> w1276
          tunnel: w1275 -> [w1285]
          tunnel: [w1290] -> w1282
          tunnel: w1281 -> [w1290]
          tunnel: [w1289] -> w1280
          tunnel: w1279 -> [w1289]
          tunnel: w1276 -> [w1288]
          tunnel: [w1311] -> w1278
          tunnel: w1282 -> [w1322]
          tunnel: w1280 -> [w1319]
          tunnel: [w1291] -> w1277
          frame #0 {
            n679 = call "Loop Timer15"("Count(Ticks)"=w1286) -> ("Tick Count(Ticks)"=w1287:u16)
          }
          frame #1 {
            # "Signal maybe then sent through \na transistor before APD"
            n680 = xnode "FPGA I/O Node"("Connector0/DIO12"=w1288, "Connector0/DIO13"=w1288, "Connector0/DIO14"=w1288, "Connector0/DIO15"=w1288) -> ()  [unwired: 4 in, 4 out]
            "APD3 int gate" <- w1288
          }
          frame #2 {
            n681 = local read "APD Gate OFF Count"() -> (w1296:u16)
            n682 = local read "APD Gate ON Count"() -> (w1297:u16)
            n683 = feedback #54(TRUE) -> (w1316:bool)
            n684 = feedback-in #55(w1322) -> ()
            n685 = feedback #55(w1322) -> (w1321:u16)
            n686 = Not(x=w1316) -> (.not. x?=w1314:bool)
            n687 = feedback-in #54(w1314) -> ()
            n688 = Subtract(x=w1322, y=w1321) -> (x-y=w1320:u16)
            n689 = Select(t=w1297, s=w1314, f=w1296) -> (s? t:f=w1318:u16)
            n690 = Subtract(x=w1320, y=w1319) -> (x-y=w1299:u16)
            n691 = Subtract(x=w1318, y=w1299) -> (x-y=w1310:u16)
            n692 = Number To Boolean Array(number=w1299) -> (Boolean array=w1300:bool[])
            n693 = Or Array Elements(Boolean array=w1300) -> (logical OR=w1298:bool)
            n694 = Boolean To (0,1)(Boolean=w1298) -> (0, 1=w1305:i16)
            n695 = Boolean To (0,1)(Boolean="+ phase (APD 3 Gate)") -> (0, 1=w1308:i16)
            n696 = To Unsigned Byte Integer(number=w1305) -> (unsigned 8bit integer=w1302:u8)
            n697 = Multiply(x=w1308, y="Phase count adjustment (APD 3 Gate)") -> (x*y=w1306:i16)
            n698 = feedback #56(u8 0) -> (w1303:u8)
            n699 = Add(x=w1302, y=w1303) -> (x+y=w1301:u8)
            "APD 3 Gate Late Counter" <- w1301
            n700 = feedback-in #56(w1301) -> ()
            n701 = Add(x=w1310, y=w1306) -> (x+y=w1311:u16)
            n702 = feedback #57(i16 0) -> (w1313:i16)
            n703 = Subtract(x=w1313, y=w1306) -> (x-y=w1312:i16)
            "APD 3 Gate Relative Phase" <- w1312
            n704 = feedback-in #57(w1312) -> ()
            n705 = local read "APD Gate Operating Mode"() -> (w1295:u8)
            n706 = case shown="2" w1295 {
              tunnel: [TRUE FALSE w1325] -> w1292
              tunnel: w1316 -> [_ _ w1325]
              frame 0, Default {
              }
              frame 1 {
              }
              frame 2 {
              }
            }
            n707 = local read "Invert APD Gate"() -> (w1294:bool)
            n708 = Not(x=w1292) -> (.not. x?=w1293:bool)
            n709 = Select(t=w1293, s=w1294, f=w1292) -> (s? t:f=w1291:bool)
          }
        }
      }
    }
    frame Enabled {
    }
  }
  n710 = disable-structure shown="Disabled" {
    disable-tunnel: w5 -> [w1327 _]
    disable-tunnel: w4 -> [w1326 _]
    frame Disabled {
      n711 = while "633 nm red  fluorescent laser interlacing (DO to IA 633 nm AOM ME amp)." {
        shift-right: [w1331] -> _
        shift-left: w1326 -> [w1336]
        shift-right: [w1330] -> _
        shift-left: w1327 -> [w1328]
        stop <- FALSE stop-if-true
        n712 = flat-sequence {
          tunnel: w1336 -> [w1339]
          tunnel: [w1340] -> w1334
          tunnel: [w1339] -> w1332
          tunnel: [w1338] -> w1329
          tunnel: w1328 -> [w1338]
          tunnel: [w1343] -> w1335
          tunnel: w1334 -> [w1343]
          tunnel: [w1342] -> w1333
          tunnel: w1332 -> [w1342]
          tunnel: w1329 -> [w1341]
          tunnel: [w1352] -> w1331
          tunnel: w1335 -> [w1372]
          tunnel: w1333 -> [w1369]
          tunnel: [w1361] -> w1330
          frame #0 {
            n713 = call "Loop Timer11"("Count(Ticks)"=w1339) -> ("Tick Count(Ticks)"=w1340:u16)
          }
          frame #1 {
            # "Then to PRL 440 amp"
            n714 = xnode "FPGA I/O Node"("Connector1/DIO32"=w1341) -> ()  [unwired: 1 in, 1 out]
          }
          frame #2 {
            n715 = feedback-in #58(w1372) -> ()
            n716 = feedback #58(w1372) -> (w1371:u16)
            n717 = Subtract(x=w1372, y=w1371) -> (x-y=w1370:u16)
            n718 = Subtract(x=w1370, y=w1369) -> (x-y=w1345:u16)
            n719 = Number To Boolean Array(number=w1345) -> (Boolean array=w1346:bool[])
            n720 = Or Array Elements(Boolean array=w1346) -> (logical OR=w1344:bool)
            n721 = Boolean To (0,1)(Boolean="+ phase (RI)") -> (0, 1=w1357:i16)
            n722 = Multiply(x=w1357, y="Phase count adjustment (RI)") -> (x*y=w1354:i16)
            n723 = Boolean To (0,1)(Boolean=w1344) -> (0, 1=w1351:i16)
            n724 = To Unsigned Byte Integer(number=w1351) -> (unsigned 8bit integer=w1348:u8)
            n725 = feedback #59(i16 0) -> (w1355:i16)
            n726 = feedback #60(u8 0) -> (w1349:u8)
            n727 = Add(x=w1348, y=w1349) -> (x+y=w1347:u8)
            "RI Late Counter" <- w1347
            n728 = feedback-in #60(w1347) -> ()
            n729 = Subtract(x=w1355, y=w1354) -> (x-y=w1353:i16)
            "RI Relative phase" <- w1353
            n730 = feedback-in #59(w1353) -> ()
            n731 = feedback #61(TRUE) -> (w1364:bool)
            n732 = case shown="2" "Red Laser Operating Mode" {
              tunnel: [TRUE FALSE w1378] -> w1361
              tunnel: w1364 -> [_ _ w1375]
              frame 0, Default {
              }
              frame 1 {
              }
              frame 2 {
                n733 = Not(x=w1375) -> (.not. x?=w1377:bool)
                n734 = Select(t=w1377, s="Invert RI", f=w1375) -> (s? t:f=w1378:bool)
              }
            }
            n735 = Not(x=w1364) -> (.not. x?=w1360:bool)
            n736 = Select(t="Red interlace ON count", s=w1360, f="Red interlace OFF count") -> (s? t:f=w1366:u16)
            n737 = Subtract(x=w1366, y=w1345) -> (x-y=w1358:u16)
            n738 = Add(x=w1358, y=w1354) -> (x+y=w1352:u16)
            n739 = feedback-in #61(w1360) -> ()
          }
        }
      }
    }
    frame Enabled {
    }
  }
  n740 = disable-structure shown="Disabled" {
    disable-tunnel: w4 -> [w1379 _]
    frame Disabled {
      n741 = while "Blue fluorescent laser interlacing (AO control direct to laser)." {
        shift-right: [w1386] -> _
        shift-left: w1379 -> [w1389]
        shift-right: [w1383] -> _
        shift-left: i16 0 -> [w1381]
        stop <- FALSE stop-if-true
        n742 = flat-sequence {
          tunnel: w1389 -> [w1392]
          tunnel: [w1393] -> w1388
          tunnel: [w1392] -> w1387
          tunnel: [w1391] -> w1382
          tunnel: w1381 -> [w1391]
          tunnel: [w1396] -> w1385
          tunnel: w1388 -> [w1396]
          tunnel: [w1395] -> w1384
          tunnel: w1387 -> [w1395]
          tunnel: w1382 -> [w1394]
          tunnel: [w1406] -> w1386
          tunnel: [w1422] -> w1383
          tunnel: w1385 -> [w1434]
          tunnel: w1384 -> [w1431]
          frame #0 {
            n743 = call "Loop Timer13"("Count(Ticks)"=w1392) -> ("Tick Count(Ticks)"=w1393:u16)
          }
          frame #1 {
            n744 = xnode "FPGA I/O Node"("Connector0/AO3"=w1394) -> ()  [unwired: 1 in, 1 out]
          }
          frame #2 {
            n745 = Subtract(x="Blue OFF count (AO)", y="Blue current ON count adj (AO)") -> (x-y=w1415:u16)
            n746 = feedback-in #62(w1434) -> ()
            n747 = feedback #62(w1434) -> (w1433:u16)
            n748 = Add(x="Blue current ON count adj (AO)", y="Blue ON count (AO)") -> (x+y=w1416:u16)
            n749 = Subtract(x=w1434, y=w1433) -> (x-y=w1432:u16)
            n750 = Subtract(x=w1432, y=w1431) -> (x-y=w1399:u16)
            n751 = Number To Boolean Array(number=w1399) -> (Boolean array=w1400:bool[])
            n752 = Boolean To (0,1)(Boolean="+ phase (BI AO)") -> (0, 1=w1412:i16)
            n753 = Or Array Elements(Boolean array=w1400) -> (logical OR=w1398:bool)
            n754 = Boolean To (0,1)(Boolean=w1398) -> (0, 1=w1405:i16)
            n755 = Multiply(x=w1412, y="Phase count adjustment (BI AO)") -> (x*y=w1408:i16)
            n756 = To Unsigned Byte Integer(number=w1405) -> (unsigned 8bit integer=w1401:u8)
            n757 = feedback #63(u8 0) -> (w1403:u8)
            n758 = Add(x=w1401, y=w1403) -> (x+y=w1402:u8)
            "BI Late Counter (AO)" <- w1402
            n759 = feedback-in #63(w1402) -> ()
            n760 = feedback #64(i16 0) -> (w1409:i16)
            n761 = Subtract(x=w1409, y=w1408) -> (x-y=w1407:i16)
            "BI Relative phase (AO)" <- w1407
            n762 = feedback-in #64(w1407) -> ()
            n763 = feedback #65(TRUE) -> (w1426:bool)
            n764 = case shown="2" "BI Operating Mode (AO)" {
              tunnel: [TRUE FALSE w1450] -> w1417
              tunnel: w1426 -> [_ _ w1447]
              frame 0, Default {
              }
              frame 1 {
              }
              frame 2 {
                n765 = Not(x=w1447) -> (.not. x?=w1449:bool)
                n766 = Select(t=w1449, s="Invert BI (AO)", f=w1447) -> (s? t:f=w1450:bool)
              }
            }
            n767 = And(x=w1417, y="Blue FB On/Off") -> (x .and. y?=w1418:bool)
            n768 = case shown="True" w1418 {
              tunnel: "BI Current Out" -> [w1435 _]
              tunnel: [w1435 w1437] -> w1421
              frame False {
              }
              frame True {
                n769 = local read "Blue Intensity"() -> (w1436:i16)
                n770 = Bundle("P5"="P5", "I5"="I5", "D5"="D5") -> (w1438:cluster{"P5":i16, "I5":i16, "D5":i16})  [unwired: 1 in]
                n771 = call "Slower PID.vi"("process variable"=w1436, "reset?"="Blue FB Reset", "setpoint"="Blue FB Setpoint", "PID gains (x 2^8)"=w1438, "output range"=cluster{"output high":i16, "output low":i16} {"output high"=32767, "output low"=0} ("Green FB output range")) -> ("output"=w1437:i16)  [unwired: 10 out]
              }
            }
            n772 = Not(x=w1426) -> (.not. x?=w1423:bool)
            n773 = Select(t=w1416, s=w1423, f=w1415) -> (s? t:f=w1428:u16)
            n774 = Subtract(x=w1428, y=w1399) -> (x-y=w1410:u16)
            n775 = Add(x=w1410, y=w1408) -> (x+y=w1406:u16)
            n776 = feedback-in #65(w1423) -> ()
            n777 = Boolean To (0,1)(Boolean=w1417) -> (0, 1=w1397:i16)
            n778 = Multiply(x=w1397, y=w1421) -> (x*y=w1422:i16)
          }
        }
      }
    }
    frame Enabled {
    }
  }
  n779 = disable-structure shown="Disabled" {
    disable-tunnel: w5 -> [w1452 _]
    disable-tunnel: w4 -> [w1451 _]
    frame Disabled {
      n780 = while "473 nm blue  fluorescent laser interlacing (DO to blue laser digital control input)." {
        shift-right: [w1456] -> _
        shift-left: w1451 -> [w1461]
        shift-right: [w1455] -> _
        shift-left: w1452 -> [w1453]
        stop <- FALSE stop-if-true
        n781 = flat-sequence {
          tunnel: w1461 -> [w1464]
          tunnel: [w1465] -> w1459
          tunnel: [w1464] -> w1457
          tunnel: [w1463] -> w1454
          tunnel: w1453 -> [w1463]
          tunnel: [w1468] -> w1460
          tunnel: w1459 -> [w1468]
          tunnel: [w1467] -> w1458
          tunnel: w1457 -> [w1467]
          tunnel: w1454 -> [w1466]
          tunnel: [w1477] -> w1456
          tunnel: w1460 -> [w1497]
          tunnel: w1458 -> [w1494]
          tunnel: [w1486] -> w1455
          frame #0 {
            n782 = call "Loop Timer14"("Count(Ticks)"=w1464) -> ("Tick Count(Ticks)"=w1465:u16)
          }
          frame #1 {
            n783 = xnode "FPGA I/O Node"("Connector1/DIO28"=w1466) -> ()  [unwired: 1 in, 1 out]
          }
          frame #2 {
            n784 = feedback-in #66(w1497) -> ()
            n785 = feedback #66(w1497) -> (w1496:u16)
            n786 = Subtract(x=w1497, y=w1496) -> (x-y=w1495:u16)
            n787 = Subtract(x=w1495, y=w1494) -> (x-y=w1470:u16)
            n788 = Number To Boolean Array(number=w1470) -> (Boolean array=w1471:bool[])
            n789 = Or Array Elements(Boolean array=w1471) -> (logical OR=w1469:bool)
            n790 = Boolean To (0,1)(Boolean="+ phase (BI D)") -> (0, 1=w1482:i16)
            n791 = Multiply(x=w1482, y="Phase count adjustment (BI D)") -> (x*y=w1479:i16)
            n792 = Boolean To (0,1)(Boolean=w1469) -> (0, 1=w1476:i16)
            n793 = To Unsigned Byte Integer(number=w1476) -> (unsigned 8bit integer=w1473:u8)
            n794 = feedback #67(i16 0) -> (w1480:i16)
            n795 = feedback #68(u8 0) -> (w1474:u8)
            n796 = Add(x=w1473, y=w1474) -> (x+y=w1472:u8)
            "Blue Late Counter (D)" <- w1472
            n797 = feedback-in #68(w1472) -> ()
            n798 = Subtract(x=w1480, y=w1479) -> (x-y=w1478:i16)
            "BI Relative phase (D)" <- w1478
            n799 = feedback-in #67(w1478) -> ()
            n800 = feedback #69(TRUE) -> (w1489:bool)
            n801 = case shown="2" "Blue Laser Operating Mode (D)" {
              tunnel: [TRUE FALSE w1503] -> w1486
              tunnel: w1489 -> [_ _ w1500]
              frame 0, Default {
              }
              frame 1 {
              }
              frame 2 {
                n802 = Not(x=w1500) -> (.not. x?=w1502:bool)
                n803 = Select(t=w1502, s="Invert BI (D)", f=w1500) -> (s? t:f=w1503:bool)
              }
            }
            n804 = Not(x=w1489) -> (.not. x?=w1485:bool)
            n805 = Select(t="Blue interlace ON count (D)", s=w1485, f="Blue interlace OFF count (D)") -> (s? t:f=w1491:u16)
            n806 = Subtract(x=w1491, y=w1470) -> (x-y=w1483:u16)
            n807 = Add(x=w1483, y=w1479) -> (x+y=w1477:u16)
            n808 = feedback-in #69(w1485) -> ()
          }
        }
      }
    }
    frame Enabled {
    }
  }
